vi "FPGA Main Default.vi"() -> ()   [LabVIEW 2019]
uses:
  Sub VIs/Utilities/Start Boolean.ctl
  <vilib>/Platform/TimedLoop/XDataNode/timing_clust.ctl
  <vilib>/Platform/TimedLoop/XDataNode/nitl_modes.ctl
  <vilib>/Platform/TimedLoop/XDataNode/wakeup.ctl
  Sub VIs/Utilities/SPI Configuration Group.ctl
  Sub VIs/Utilities/I2C Configuration Group.ctl
  Sub VIs/Utilities/PWM Configuration Group.ctl
  Sub VIs/Utilities/Encoder Configuration Group.ctl
  <vilib>/rvi/Emulation/niFpgaGetClockAttributes.vi
  <vilib>/rvi/Emulation/niFpgaSctlEmulationGetInTimedLoop.vi
  <vilib>/rvi/Emulation/niFpgaEmulationReportErrorSimple.vi
  <vilib>/rvi/Emulation/niFpgaEmulationIsFPGAContextNoSignature.vi
  <vilib>/rvi/errors/niFpgaSetErrorForExecOnDevCompSimple.vi
  <vilib>/rvi/eio/common/nirviEmuReportErrorAndStop.vi
  <vilib>/rvi/DataTransferAndStorage/Container/Common/niFpgaContainerGetUniqueNameForEmu.vi
  <vilib>/rvi/FIFO/Fifo_Resource/nirvififoEmulationSetSize.vi
  <vilib>/rvi/FIFO/Fifo_Resource/nirviFifoEmulationQueueMgr.vi
  <instcachedir>/0/nirviFifoEmulationQueueMgr_E5CAEC123FF24DC58D834DCA3CDAA9B5.lvgen/nirviFifoEmulationQueueMgr_E5CAEC123FF24DC58D834DCA3CDAA9B5_003.vi
  <vilib>/Utility/error.llb/Clear Errors.vi
  <vilib>/rvi/FIFO/Fifo_Resource/nirvififoEmulationCreateLock.vi
  <vilib>/rvi/Emulation/niFpgaProcessEmulError.vi
  <vilib>/rvi/FIFO/Fifo_Resource/nirvififoEmulationObtainLock.vi
  <vilib>/rvi/FIFO/Fifo_Resource/nirvififoEmulationReleaseLock.vi
  <vilib>/rvi/occurrence/nirviWaitOnOccurrenceBase.vi
  <vilib>/rvi/errors/nirviReportUnexpectedCaseInternalError.vi
  <vilib>/rvi/errors/nirviReportUnexpectedCaseInternalError (U32).vi
  <vilib>/rvi/FIFO/Fifo_Resource/nirvififoEmulationDetermineInputValidOut.vi
  <vilib>/rvi/Emulation/niFpgaCriticalErrorInLSC.vi
  <instcachedir>/0/nirviFifoEmulationQueueMgr_E5CAEC123FF24DC58D834DCA3CDAA9B5.lvgen/nirviFifoEmulationQueueMgr_E5CAEC123FF24DC58D834DCA3CDAA9B5_004.vi
  <instcachedir>/0/nirviFifoEmulationQueueMgr_E5CAEC123FF24DC58D834DCA3CDAA9B5.lvgen/nirviFifoEmulationQueueMgr_E5CAEC123FF24DC58D834DCA3CDAA9B5_005.vi
  <vilib>/rvi/eio/common/nirviEmuTemplateMethod_errors.vi
  <vilib>/rvi/interface/RandomDataEmulation/niFpgaRandomDataHandleErrors.vi
  Sub VIs/Utilities/ELVIS III Global.vi
  <vilib>/rvi/eio/common/nirviEmuTemplatePropertyGet_noerrors.vi
  <vilib>/rvi/eio/common/nirviEmuTemplatePropertySet_noerrors.vi
  <vilib>/rvi/Memory/Memory_Emulation/niFpgaMemoryEmulationCacheClearOnFirstRun.vi
  <vilib>/rvi/Memory/Memory_Emulation/nirvimemoryEmulationManagerCache_MakeExclusive.vi
  <vilib>/rvi/Memory/Memory_Emulation/niFpgaMemoryEmulationValidateCache.vi
  <vilib>/rvi/Memory/Memory_Emulation/nirvimemoryEmulationManagerCache_InsertValue.vi
  <vilib>/rvi/Memory/Memory_Emulation/nirvimemoryEmulationManagerCache_ReleaseExclusive.vi
  <vilib>/rvi/Memory/Memory_Emulation/nirvimemoryEmulationManagerCache_GetValue.vi
  <vilib>/rvi/Memory/Memory_Emulation/nirvimemoryEmulationManagerCache_SetValue.vi
  <vilib>/rvi/Memory/Memory_Emulation/nirvimemoryFastEmulation.vi
  <vilib>/rvi/Memory/Memory_Emulation/nirvimemoryEmulation.vi
  <vilib>/rvi/DataTransferAndStorage/Container/Common/niFpgaContainerSetEmuInfo.vi
  <vilib>/rvi/DataTransferAndStorage/Container/XNode/niFpgaContainer.xnode
  <vilib>/rvi/FIFO/Fifo_Resource/nirvififoEmulationRead.vi
  <vilib>/rvi/FIFO/Fifo_Resource/nirvififoEmulationWrite.vi
  <vilib>/Platform/TimedLoop/XDataNode/XDataNode.xnode
  <vilib>/eio/EIOMethodNode/EIOMethodNode.xnode
  <vilib>/LabVIEW Targets/FPGA/RIO/BlueMoonOnboardIO/nicrio_cRIO-BlueMoonOnboardAi_VoltageRange.ctl
  <vilib>/LabVIEW Targets/FPGA/RIO/BlueMoonOnboardIO/nicrio_cRIO-BlueMoonOnboardAi_TerminalMod.ctl
  <vilib>/rvi/interface/RandomDataEmulation/nirviRandomDataFpgaReadWriteTemplate.vi
  <vilib>/eio/EIOPropertyNode/EIOPropertyNode.xnode
  <vilib>/eio/EIONode/EIONode.xnode
  <vilib>/rvi/DataTransferAndStorage/Register/Emulation/niFpgaRegisterEmulation.vi
  <vilib>/rvi/LocalResourceManager/LocalResourceManager.xnode
  <vilib>/Platform/TimedLoop/XDataNode/XDNodeRunTimeDep.lvlib
  <vilib>/rvi/eio/common/nirviEmuTemplatePropertyGet_errors.vi
  <vilib>/rvi/eio/common/nirviEmuTemplatePropertySet_errors.vi
panel:
  in  "DATAGEN.B_1.CNTR":u32
  in  "DATAGEN.B_0.CNTR":u32
  in  "DATAGEN.A_1.CNTR":u32
  in  "DATAGEN.A_0.CNTR":u32
  in  "DATAGEN.ENA":fxp<+,4,4>
  in  "DATAGEN.A_0.FREQ_DIV":fxp<+,32,0>
  in  "DATAGEN.A_1.FREQ_DIV":fxp<+,32,0>
  in  "DATAGEN.B_1.FREQ_DIV":fxp<+,32,0>
  in  "DATAGEN.B_0.FREQ_DIV":fxp<+,32,0>
  out "DMA.SYS.RDY":bool
  out "AO.B.ELE_NUM":u32
  out "AO.A.ELE_NUM":u32
  in  "AO.B.SYNC":T1
  in  "AO.A.SYNC":T1
  in  "AO.SYNC":T1
  in  "SYNC":T1
  in  "B.SYNC":T1
  in  "A.SYNC":T1
  out "AI.A.STAT":u8
  out "AI.B.STAT":u8
  out "AI.DIFF_B_3.VAL":fxp<+/-,26,5>
  out "AI.DIFF_B_2.VAL":fxp<+/-,26,5>
  out "AI.DIFF_B_1.VAL":fxp<+/-,26,5>
  out "AI.DIFF_B_0.VAL":fxp<+/-,26,5>
  out "AI.B_7.VAL":fxp<+/-,26,5>
  out "AI.B_6.VAL":fxp<+/-,26,5>
  out "AI.B_5.VAL":fxp<+/-,26,5>
  out "AI.B_4.VAL":fxp<+/-,26,5>
  out "AI.B_3.VAL":fxp<+/-,26,5>
  out "AI.B_2.VAL":fxp<+/-,26,5>
  out "AI.B_1.VAL":fxp<+/-,26,5>
  out "AI.B_0.VAL":fxp<+/-,26,5>
  out "AI.DIFF_A_3.VAL":fxp<+/-,26,5>
  out "AI.DIFF_A_2.VAL":fxp<+/-,26,5>
  out "AI.DIFF_A_1.VAL":fxp<+/-,26,5>
  out "AI.DIFF_A_0.VAL":fxp<+/-,26,5>
  out "AI.A_7.VAL":fxp<+/-,26,5>
  out "AI.A_6.VAL":fxp<+/-,26,5>
  out "AI.A_5.VAL":fxp<+/-,26,5>
  out "AI.A_4.VAL":fxp<+/-,26,5>
  out "AI.A_3.VAL":fxp<+/-,26,5>
  out "AI.A_2.VAL":fxp<+/-,26,5>
  out "AI.A_1.VAL":fxp<+/-,26,5>
  out "AI.A_0.VAL":fxp<+/-,26,5>
  in  "UART.A.ENA":bool
  in  "UART.B.ENA":bool
  out "CONSOLE.ENA":bool
  in  "DO.LED3:0":u8 format="%04b"
  out "DI.BTN":u8 format="%08b"
  in  "IRQ.DI_BTN.ENA":bool
  in  "IRQ.DI_BTN.RISE":bool
  in  "IRQ.DI_BTN.FALL":bool
  in  "IRQ.DI_BTN.CNT":u32
  in  "IRQ.DI_BTN.NO":u8
  in  "IRQ.AI_A_1.NO":u8
  in  "IRQ.AI_A_0.NO":u8
  in  "IRQ.AI_A_1.THRESHOLD":fxp<+/-,26,5>
  in  "IRQ.AI_A_0.THRESHOLD":fxp<+/-,26,5>
  in  "IRQ.AI_A.CNFG":u8 format="%.0b"
  in  "IRQ.AI_A_0.HYSTERESIS":fxp<+/-,26,5>=15.999999523162842
  in  "IRQ.AI_A_1.HYSTERESIS":fxp<+/-,26,5>=15.999999523162842
  in  "IRQ.DIO_A_3.NO":u8
  in  "IRQ.DIO_A_2.NO":u8
  in  "IRQ.DIO_A_1.NO":u8
  in  "IRQ.DIO_A_0.NO":u8
  in  "IRQ.DIO_A_3.CNT":u32
  in  "IRQ.DIO_A_2.CNT":u32
  in  "IRQ.DIO_A_1.CNT":u32
  in  "IRQ.DIO_A_0.CNT":u32
  in  "IRQ.DIO_A_7:0.FALL":u8 format="%08b"
  in  "IRQ.DIO_A_7:0.RISE":u8 format="%08b"
  in  "IRQ.DIO_A_7:0.ENA":u8 format="%08b"
  in  "IRQ.TIMER.SETTIME":T1
  in  "IRQ.TIMER.WRITE":u32
  out "IRQ.TIMER.READ":u32
  out "UART.B.STAT":bool
  out "UART.A.STAT":bool
  out "AI.B.DMA_FULL":bool
  in  "AI.B.DMA_ENA":bool
  out "AI.B.VAL.RDY":bool
  in  "AI.B.CNFG":u8[](array[numeric])=[0, 1, 2, 3, 4, 5, 6, 7, 0, 0, 0, 0] format="%.0x"
  in  "AI.B.CNT":u8
  in  "AI.B.CNTR":u32=2000
  out "AO.B.DMA_IDL":bool
  in  "AO.B.DMA_CNTR":u32=200
  out "AO.A.DMA_IDL":bool
  in  "AO.A.DMA_CNTR":u32=200
  in  "AI.A.DMA_ENA":bool
  out "AI.A.DMA_FULL":bool
  out "AI.A.VAL.RDY":bool
  in  "AI.A.CNT":u8
  in  "AI.A.CNTR":u32=2000
  in  "AI.A.CNFG":u8[](array[numeric])=[0, 1, 2, 3, 4, 5, 6, 7, 0, 0, 0, 0] format="%.0x"
  in  "AO.B.DMA_ENA":fxp<+,2,2> format="%04b"
  out "AO.SYS.STAT":bool
  in  "AO.A.DMA_ENA":fxp<+,2,2> format="%04b"
  in  "AO.SYS.GO":T1
  in  "AO.B_0.VAL":fxp<+/-,20,5> format="%#_17g"
  in  "AO.B_1.VAL":fxp<+/-,20,5> format="%#_17g"
  in  "AO.A_0.VAL":fxp<+/-,20,5> format="%#_17g"
  in  "AO.A_1.VAL":fxp<+/-,20,5> format="%#_17g"
  in  "DIO.B_19:0.DIR":fxp<+,20,20> format="%.0b"
  in  "DO.B.DMA_CNTR":u16 format="%.0b"
  out "DIO.B_19:0.IN":fxp<+,20,20> format="%.0b"
  out "DI.B.DMA_IDL":bool
  in  "DIO.B_19:0.OUT":fxp<+,20,20> format="%.0b"
  out "DO.B.DMA_IDL":bool
  in  "DO.B.DMA_ENA":fxp<+,20,20> format="%020b"
  in  "DI.B.DMA_ENA":bool
  in  "DI.B.DMA_CNTR":u16 format="%.0b"
  in  "SYS.SELECTB":u64 format="%010x"
  out "ENC.B_0.CNTR":u32
  out "ENC.B_0.STAT":u8 format="%08b"
  in  "ENC.B_0.CNFG":u8
  in  "PWM.B_0.MAX":u16
  in  "PWM.B_0.CMP":u16
  in  "PWM.B_0.CNFG":u8 format="%08b"
  in  "PWM.B_0.CS":u8
  in  "PWM.B_1.MAX":u16
  in  "PWM.B_1.CMP":u16
  in  "PWM.B_1.CNFG":u8 format="%08b"
  in  "PWM.B_1.CS":u8
  out "PWM.B_0.CNTR":u16
  out "PWM.B_1.CNTR":u16
  in  "PWM.B_2.MAX":u16
  in  "PWM.B_2.CMP":u16
  in  "PWM.B_2.CNFG":u8 format="%08b"
  in  "PWM.B_2.CS":u8
  in  "PWM.B_3.MAX":u16
  in  "PWM.B_3.CMP":u16
  in  "PWM.B_3.CNFG":u8 format="%08b"
  in  "PWM.B_3.CS":u8
  in  "ENC.B_1.CNFG":u8
  out "ENC.B_1.CNTR":u32
  out "ENC.B_1.STAT":u8 format="%08b"
  out "PWM.B_2.CNTR":u16
  out "PWM.B_3.CNTR":u16
  in  "PWM.B_4.MAX":u16
  in  "PWM.B_4.CMP":u16
  in  "PWM.B_4.CNFG":u8 format="%08b"
  in  "PWM.B_4.CS":u8
  in  "PWM.B_5.MAX":u16
  in  "PWM.B_5.CMP":u16
  in  "PWM.B_5.CNFG":u8 format="%08b"
  in  "PWM.B_5.CS":u8
  in  "PWM.B_6.MAX":u16
  in  "PWM.B_6.CMP":u16
  in  "PWM.B_6.CNFG":u8 format="%08b"
  in  "PWM.B_6.CS":u8
  in  "PWM.B_7.MAX":u16
  in  "PWM.B_7.CMP":u16
  in  "PWM.B_7.CNFG":u8 format="%08b"
  in  "PWM.B_7.CS":u8
  out "ENC.B_2.CNTR":u32
  out "ENC.B_2.STAT":u8 format="%08b"
  out "PWM.B_4.CNTR":u16
  out "PWM.B_5.CNTR":u16
  out "PWM.B_6.CNTR":u16
  out "PWM.B_7.CNTR":u16
  out "ENC.B_3.CNTR":u32
  out "ENC.B_3.STAT":u8 format="%08b"
  in  "ENC.B_2.CNFG":u8
  in  "ENC.B_3.CNFG":u8
  out "SPI.B.STAT":u8 format="%08b"
  in  "SPI.B.GO":T1
  in  "SPI.B.CNT":u16=19
  in  "SPI.B.CNFG":u16=112
  out "SPI.B.DATI":u16
  in  "SPI.B.DATO":u16
  out "ENC.B_4.CNTR":u32
  out "ENC.B_4.STAT":u8 format="%08b"
  in  "ENC.B_4.CNFG":u8
  in  "PWM.B_8.MAX":u16
  in  "PWM.B_8.CMP":u16
  in  "PWM.B_8.CNFG":u8 format="%08b"
  in  "PWM.B_8.CS":u8
  in  "PWM.B_9.MAX":u16
  in  "PWM.B_9.CMP":u16
  in  "PWM.B_9.CNFG":u8 format="%08b"
  in  "PWM.B_9.CS":u8
  out "PWM.B_8.CNTR":u16
  out "PWM.B_9.CNTR":u16
  out "ENC.B_5.CNTR":u32
  out "ENC.B_5.STAT":u8 format="%08b"
  in  "ENC.B_5.CNFG":u8
  in  "PWM.B_10.MAX":u16
  in  "PWM.B_10.CMP":u16
  in  "PWM.B_10.CNFG":u8 format="%08b"
  in  "PWM.B_10.CS":u8
  in  "PWM.B_11.MAX":u16
  in  "PWM.B_11.CMP":u16
  in  "PWM.B_11.CNFG":u8 format="%08b"
  in  "PWM.B_11.CS":u8
  out "PWM.B_10.CNTR":u16
  out "PWM.B_11.CNTR":u16
  out "ENC.B_6.CNTR":u32
  out "ENC.B_6.STAT":u8 format="%08b"
  in  "ENC.B_6.CNFG":u8
  in  "PWM.B_12.MAX":u16
  in  "PWM.B_12.CMP":u16
  in  "PWM.B_12.CNFG":u8 format="%08b"
  in  "PWM.B_12.CS":u8
  in  "PWM.B_13.MAX":u16
  in  "PWM.B_13.CMP":u16
  in  "PWM.B_13.CNFG":u8 format="%08b"
  in  "PWM.B_13.CS":u8
  out "PWM.B_12.CNTR":u16
  out "PWM.B_13.CNTR":u16
  out "ENC.B_7.CNTR":u32
  out "ENC.B_7.STAT":u8 format="%08b"
  in  "ENC.B_7.CNFG":u8
  in  "PWM.B_14.MAX":u16
  in  "PWM.B_14.CMP":u16
  in  "PWM.B_14.CNFG":u8 format="%08b"
  in  "PWM.B_14.CS":u8
  in  "PWM.B_15.MAX":u16
  in  "PWM.B_15.CMP":u16
  in  "PWM.B_15.CNFG":u8 format="%08b"
  in  "PWM.B_15.CS":u8
  out "PWM.B_14.CNTR":u16
  out "PWM.B_15.CNTR":u16
  in  "I2C.B.GO":T1
  in  "I2C.B.CNFG":u8=1 format="%08b"
  in  "I2C.B.DATO":u8
  out "I2C.B.DATI":u8
  in  "I2C.B.ADDR":u8 format="%08b"
  in  "I2C.B.CNTR":u8=213
  in  "I2C.B.CNTL":u8 format="%08b"
  out "I2C.B.STAT":u8 format="%08b"
  out "ENC.B_8.CNTR":u32
  out "ENC.B_8.STAT":u8 format="%08b"
  in  "ENC.B_8.CNFG":u8
  in  "PWM.B_16.MAX":u16
  in  "PWM.B_16.CMP":u16
  in  "PWM.B_16.CNFG":u8 format="%08b"
  in  "PWM.B_16.CS":u8
  in  "PWM.B_17.MAX":u16
  in  "PWM.B_17.CMP":u16
  in  "PWM.B_17.CNFG":u8 format="%08b"
  in  "PWM.B_17.CS":u8
  out "PWM.B_16.CNTR":u16
  out "PWM.B_17.CNTR":u16
  out "ENC.B_9.CNTR":u32
  out "ENC.B_9.STAT":u8 format="%08b"
  in  "ENC.B_9.CNFG":u8
  in  "PWM.B_18.MAX":u16
  in  "PWM.B_18.CMP":u16
  in  "PWM.B_18.CNFG":u8 format="%08b"
  in  "PWM.B_18.CS":u8
  in  "PWM.B_19.MAX":u16
  in  "PWM.B_19.CMP":u16
  in  "PWM.B_19.CNFG":u8 format="%08b"
  in  "PWM.B_19.CS":u8
  out "PWM.B_18.CNTR":u16
  out "PWM.B_19.CNTR":u16
  out "ENC.A_9.CNTR":u32
  out "ENC.A_9.STAT":u8 format="%08b"
  in  "ENC.A_9.CNFG":u8
  in  "PWM.A_18.MAX":u16
  in  "PWM.A_18.CMP":u16
  in  "PWM.A_18.CNFG":u8 format="%08b"
  in  "PWM.A_18.CS":u8
  in  "PWM.A_19.MAX":u16
  in  "PWM.A_19.CMP":u16
  in  "PWM.A_19.CNFG":u8 format="%08b"
  in  "PWM.A_19.CS":u8
  out "PWM.A_18.CNTR":u16
  out "PWM.A_19.CNTR":u16
  out "ENC.A_8.CNTR":u32
  out "ENC.A_8.STAT":u8 format="%08b"
  in  "ENC.A_8.CNFG":u8
  in  "PWM.A_16.MAX":u16
  in  "PWM.A_16.CMP":u16
  in  "PWM.A_16.CNFG":u8 format="%08b"
  in  "PWM.A_16.CS":u8
  in  "PWM.A_17.MAX":u16
  in  "PWM.A_17.CMP":u16
  in  "PWM.A_17.CNFG":u8 format="%08b"
  in  "PWM.A_17.CS":u8
  out "PWM.A_16.CNTR":u16
  out "PWM.A_17.CNTR":u16
  out "I2C.A.STAT":u8 format="%08b"
  in  "I2C.A.CNTL":u8 format="%08b"
  in  "I2C.A.CNTR":u8=213
  in  "I2C.A.ADDR":u8 format="%08b"
  out "I2C.A.DATI":u8
  in  "I2C.A.DATO":u8
  in  "I2C.A.CNFG":u8=1 format="%08b"
  in  "I2C.A.GO":T1
  out "ENC.A_7.CNTR":u32
  out "ENC.A_7.STAT":u8 format="%08b"
  in  "ENC.A_7.CNFG":u8
  in  "PWM.A_14.MAX":u16
  in  "PWM.A_14.CMP":u16
  in  "PWM.A_14.CNFG":u8 format="%08b"
  in  "PWM.A_14.CS":u8
  in  "PWM.A_15.MAX":u16
  in  "PWM.A_15.CMP":u16
  in  "PWM.A_15.CNFG":u8 format="%08b"
  in  "PWM.A_15.CS":u8
  out "PWM.A_14.CNTR":u16
  out "PWM.A_15.CNTR":u16
  out "ENC.A_6.CNTR":u32
  out "ENC.A_6.STAT":u8 format="%08b"
  in  "ENC.A_6.CNFG":u8
  in  "PWM.A_12.MAX":u16
  in  "PWM.A_12.CMP":u16
  in  "PWM.A_12.CNFG":u8 format="%08b"
  in  "PWM.A_12.CS":u8
  in  "PWM.A_13.MAX":u16
  in  "PWM.A_13.CMP":u16
  in  "PWM.A_13.CNFG":u8 format="%08b"
  in  "PWM.A_13.CS":u8
  out "PWM.A_12.CNTR":u16
  out "PWM.A_13.CNTR":u16
  out "ENC.A_5.CNTR":u32
  out "ENC.A_5.STAT":u8 format="%08b"
  in  "ENC.A_5.CNFG":u8
  in  "PWM.A_10.MAX":u16
  in  "PWM.A_10.CMP":u16
  in  "PWM.A_10.CNFG":u8 format="%08b"
  in  "PWM.A_10.CS":u8
  in  "PWM.A_11.MAX":u16
  in  "PWM.A_11.CMP":u16
  in  "PWM.A_11.CNFG":u8 format="%08b"
  in  "PWM.A_11.CS":u8
  out "PWM.A_10.CNTR":u16
  out "PWM.A_11.CNTR":u16
  out "ENC.A_4.CNTR":u32
  out "ENC.A_4.STAT":u8 format="%08b"
  in  "ENC.A_4.CNFG":u8
  in  "PWM.A_8.MAX":u16
  in  "PWM.A_8.CMP":u16
  in  "PWM.A_8.CNFG":u8 format="%08b"
  in  "PWM.A_8.CS":u8
  in  "PWM.A_9.MAX":u16
  in  "PWM.A_9.CMP":u16
  in  "PWM.A_9.CNFG":u8 format="%08b"
  in  "PWM.A_9.CS":u8
  out "PWM.A_8.CNTR":u16
  out "PWM.A_9.CNTR":u16
  in  "SPI.A.DATO":u16
  out "SPI.A.DATI":u16
  in  "SPI.A.CNFG":u16=112
  in  "SPI.A.CNT":u16=19
  in  "SPI.A.GO":T1
  out "SPI.A.STAT":u8 format="%08b"
  in  "ENC.A_3.CNFG":u8
  in  "ENC.A_2.CNFG":u8
  out "ENC.A_3.CNTR":u32
  out "ENC.A_3.STAT":u8 format="%08b"
  out "PWM.A_6.CNTR":u16
  out "PWM.A_7.CNTR":u16
  out "ENC.A_2.CNTR":u32
  out "ENC.A_2.STAT":u8 format="%08b"
  out "PWM.A_4.CNTR":u16
  out "PWM.A_5.CNTR":u16
  in  "PWM.A_6.MAX":u16
  in  "PWM.A_6.CMP":u16
  in  "PWM.A_6.CNFG":u8 format="%08b"
  in  "PWM.A_6.CS":u8
  in  "PWM.A_7.MAX":u16
  in  "PWM.A_7.CMP":u16
  in  "PWM.A_7.CNFG":u8 format="%08b"
  in  "PWM.A_7.CS":u8
  in  "PWM.A_4.MAX":u16
  in  "PWM.A_4.CMP":u16
  in  "PWM.A_4.CNFG":u8 format="%08b"
  in  "PWM.A_4.CS":u8
  in  "PWM.A_5.MAX":u16
  in  "PWM.A_5.CMP":u16
  in  "PWM.A_5.CNFG":u8 format="%08b"
  in  "PWM.A_5.CS":u8
  out "PWM.A_3.CNTR":u16
  out "PWM.A_2.CNTR":u16
  out "ENC.A_1.STAT":u8 format="%08b"
  out "ENC.A_1.CNTR":u32
  in  "ENC.A_1.CNFG":u8
  in  "PWM.A_3.CS":u8
  in  "PWM.A_3.CNFG":u8 format="%08b"
  in  "PWM.A_3.CMP":u16
  in  "PWM.A_3.MAX":u16
  in  "PWM.A_2.CS":u8
  in  "PWM.A_2.CNFG":u8 format="%08b"
  in  "PWM.A_2.CMP":u16
  in  "PWM.A_2.MAX":u16
  out "ENC.A_0.STAT":u8 format="%08b"
  out "ENC.A_0.CNTR":u32
  in  "ENC.A_0.CNFG":u8
  in  "PWM.A_1.MAX":u16
  in  "PWM.A_1.CMP":u16
  in  "PWM.A_1.CNFG":u8 format="%08b"
  in  "PWM.A_1.CS":u8
  out "PWM.A_1.CNTR":u16
  out "PWM.A_0.CNTR":u16
  in  "PWM.A_0.CS":u8
  in  "PWM.A_0.CNFG":u8 format="%08b"
  in  "PWM.A_0.CMP":u16
  in  "PWM.A_0.MAX":u16
  in  "SYS.SELECTA":u64 format="%010x"
  in  "DI.A.DMA_CNTR":u16 format="%.0b"
  in  "DI.A.DMA_ENA":bool
  in  "DO.A.DMA_ENA":fxp<+,20,20> format="%020b"
  out "DO.A.DMA_IDL":bool
  in  "DIO.A_19:0.OUT":fxp<+,20,20> format="%.0b"
  out "DI.A.DMA_IDL":bool
  out "DIO.A_19:0.IN":fxp<+,20,20> format="%.0b"
  in  "DO.A.DMA_CNTR":u16 format="%.0b"
  in  "DIO.A_19:0.DIR":fxp<+,20,20> format="%.0b"
  # "Connector B"
  # "System"
  # "Onboard Devices"
  # "Connector A"
  # "Buttons & LEDs"
  # "Digital I/O"
  # "PWM"
  # "Encoder"
  # "SPI Master"
  # "Analog Out"
  # "Analog In"
  # "Digital Interrupt"
  # "Digital I/O"
  # "PWM"
  # "Encoder"
  # "SPI Master"
  # "Analog Out"
  # "Analog In"
  # "Button Interrupt"
  # "Block Write AO"
  # "Block Write AO"
  # "Block Read DI"
  # "Block Read DI"
  # "I2C Master"
  # "I2C Master"
  # "Block Write DO"
  # "Block Write DO"
  # "Timer Interrupt"
  # "Data Generator"
  # "Data Generator"
  # "Analog Interrupt"
  # "IO Configuration"
  # "Console Output"
  # "IO Configuration"
  # "UART"
  # "UART"
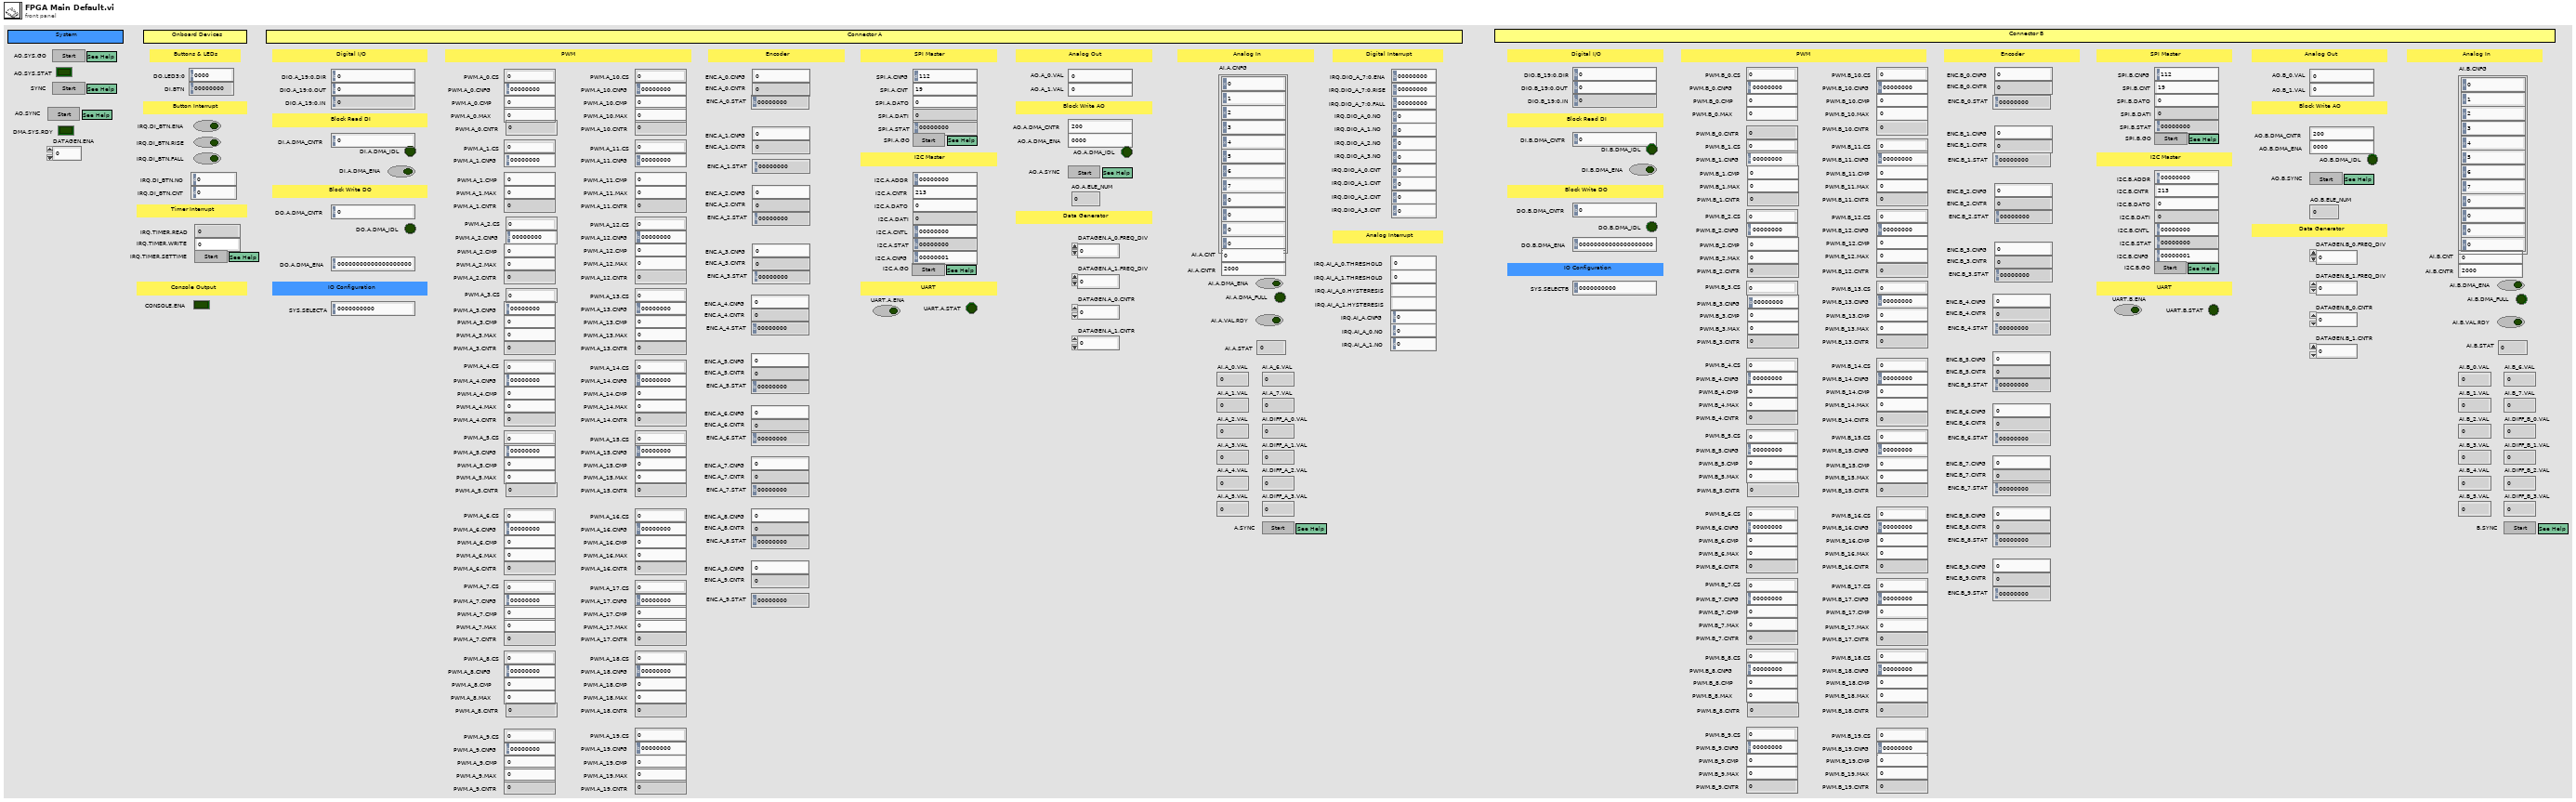
[diagram p1: front panel]
types:
  T1 = typedef "Start Boolean.ctl" = bool
  T2 = typedef "XDNodeRunTimeDep.lvlib/timing_clust.ctl" = cluster{"Expected End [f-1]":u64, "Actual End [f-1]":u64, "Finished Late? [f-1]":bool, "Expected End [i-1]":u64, "Actual End [i-1]":u64, "Finished Late? [i-1]":bool, "Expected Start [i]":u64, "Actual Start [i]":u64, "Expected Start [f]":u64, "Actual Start [f]":u64, "Source Name":string, "Structure Name":string, "Period":i64, "Deadline":i64, "Offset":i64, "Start":i64, "Priority":i32, "Timeout":i32, "Mode":T3, "Wakeup Reason":T4, "Error":errorcluster, "Source Type":string, "Secondary Source Type":string, "Global End Time":u64, "Global Start Time":u64, "Frame Duration":u64, "Iteration Duration":u64, "Assigned CPU":i32, "I/O Scan Engine Mode":u32}
  T3 = typedef "XDNodeRunTimeDep.lvlib/nitl_modes.ctl" = enum32{"No Change", "Process missed periods, maintain original phase", "Discard missed periods, maintain original phase", "Process missed periods, ignore original phase", "Discard missed periods, ignore original phase"}
  T4 = typedef "XDNodeRunTimeDep.lvlib/wakeup.ctl" = enum32{"Normal", "Aborted", "Asynchronous wakeup", "Timing source error", "Timed loop error", "Timeout"}
  T5 = typedef "Encoder Configuration Group.ctl" = cluster{"ENC.CNFG":u8, "ENC.CNTR":u32, "ENC.STAT":u8}
  T6 = typedef "PWM Configuration Group.ctl" = cluster{"PWM.0.CS":u8, "PWM.0.CNFG":u8, "PWM.0.CMP":u16, "PWM.0.MAX":u16, "PWM.0.CNTR":u16, "PWM.1.CS":u8, "PWM.1.CNFG":u8, "PWM.1.CMP":u16, "PWM.1.MAX":u16, "PWM.1.CNTR":u16}
  T7 = typedef "I2C Configuration Group.ctl" = cluster{"I2C.GO":T1, "I2C.CNFG":u8, "I2C.DATO":u8, "I2C.DATI":u8, "I2C.ADDR":u8, "I2C.CNTR":u8, "I2C.CNTL":u8, "I2C.STAT":u8}
  T8 = typedef "SPI Configuration Group.ctl" = cluster{"SPI.STAT":u8, "SPI.GO":T1, "SPI.CNT":u16, "SPI.CNFG":u16, "SPI.DATI":u16, "SPI.DATO":u16}
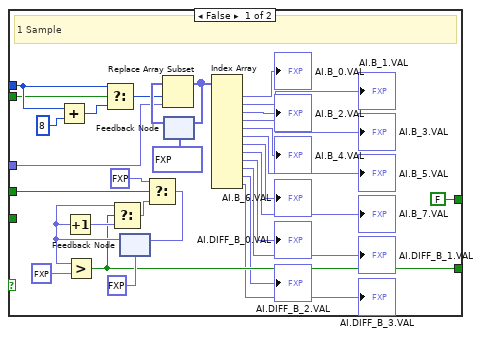
[diagram p15: hidden frame]
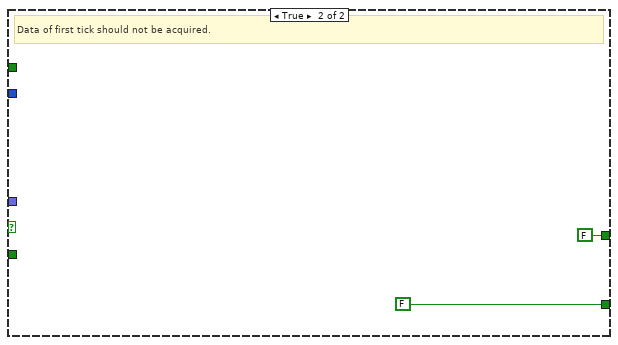
[diagram p16: hidden frame]
diagram:
  w3 = u32 0  # Address
  w4 = u32 0  # Address
  w5 = u32 0  # Address
  w6 = u32 0  # Address
  # "The Timed Loop does not allow writing the same FIFO outside the Timed Loop. Use another FIFO to push all interrupts from Button in the Timed Loop to the IRQ Queue."
  # "The FPGA timer fires the interrupt request (IRQ) when TIMER.Read counts down to zero. If TIMER.Read is not zero, it counts down to one per microsecond."
  # "The analog output nodes take some time before the FPGA write the values to the pins. The GO and STAT registers are used to handshake between the FPGA and host. When the host wants the values to be written, the host sets the GO register to TRUE. If the host reads the STAT register before setting the value of the GO register, it can wait for the value of the STAT register to invert. The value inversion tells the host that the output values have been written."
  # "The only interface that sends interrupts to the RT side. Timer interrupts, analog input interrupts, digital input interrupts, and SPI interrupt share this interface.\n\nAll interrupts work in sequence. One interrupt waits until the previous interrupt request (IRQ) gets acknowledged on the RT side."
  # "Because Write Finished Queue cannot be shared between a single-cycle Timed Loop and any other loop, Digital Write Finished Queue is required. Use this queue to transfer IRQ from DIO to IRQ Write Finished Queue."
  n1 = node-c288() -> (w8:T2)  [unwired: 1 in]
  n2 = while {
    stop <- FALSE stop-if-true
    # "Send Write Finished IRQ to RT"
    n3 = xnode ("FIFO Method Node")("超时"=-1 ("Timeout")) -> ("元素"=w25:u8)  [unwired: 1 in, 2 out]
    n4 = call <vilib>:"niFPGA Interrupt.vi"("Wait Until Cleared (F)"=TRUE, "IRQ Number (0)"=w25) -> ()  [unwired: 1 in]
  }
  n5 = timed-loop {
    timing: w8 -> [_]
    timing-out: [_] -> w7
    i -> [w29]
    stop <- _ stop-if-true
    # "DMA initialization needs 0.5s"
    n6 = Greater?(x=w29, y=20000000) -> (0:→"DMA.SYS.RDY":bool)
  }
  n7 = node-c288(w7) -> ()
  n8 = while {
    stop <- FALSE stop-if-true
    # "Timer"
    n9 = flat-sequence {
      frame #0 {
        n10 = call "Loop Timer6"("Count(uSec)"=u8 1 ("Count(mSec)")) -> ()  [unwired: 1 out]
      }
      frame #1 {
        n11 = feedback #1(u32 0 ("Timeout")) -> (w35:u32)
        n12 = Select(t="IRQ.TIMER.WRITE", s="IRQ.TIMER.SETTIME", f=w35) -> (s? t:f=w37:u32)
        n13 = case shown="默认" w37 {
          selector: w37 -> [w40 w43]
          tunnel: [w40 w41] -> w36
          frame 0 {
          }
          frame Default {
            n14 = Decrement(x=w43) -> (x-1=w42:u32)
            n15 = case shown="0" w42 {
              selector: w42 -> [w44 w47]
              tunnel: [w44 w47] -> w41
              frame Default {
              }
              frame 0 {
                n16 = global read "ELVIS III Global.vi" "Timer.IRQ_NO"() -> (w45:u8)
                n17 = xnode ("FIFO Method Node")("元素"=w45, "超时"=-1 ("Timeout")) -> ()  [unwired: 1 in, 2 out]
              }
            }
          }
        }
        "IRQ.TIMER.READ" <- w36
        n18 = feedback-in #1(w36) -> ()
      }
    }
  }
  n19 = while {
    stop <- FALSE stop-if-true
    # "DO Bank A Block Write Finished IRQ"
    n20 = feedback #2(u8 0 ("Element")) -> (w52:u8)
    n21 = feedback #3(FALSE ("Timed Out?")) -> (w54:bool)
    n22 = case shown="假" w54 {
      tunnel: [w56 w58] -> w48
      tunnel: w52 -> [_ w58]
      frame False {
        n23 = xnode ("FIFO Method Node")("超时"=-1 ("Timeout")) -> ("元素"=w56:u8)  [unwired: 1 in, 2 out]
      }
      frame True {
      }
    }
    n24 = feedback-in #2(w48) -> ()
    n25 = xnode ("FIFO Method Node")("元素"=w48, "超时"=0 ("Timeout")) -> ("超时？"=w49:bool)  [unwired: 1 in, 1 out]
    n26 = feedback-in #3(w49) -> ()
  }
  n27 = while {
    stop <- FALSE stop-if-true
    # "DO Bank B Block Write Finished IRQ"
    n28 = feedback #4(u8 0 ("Element")) -> (w63:u8)
    n29 = feedback #5(FALSE ("Timed Out?")) -> (w65:bool)
    n30 = case shown="假" w65 {
      tunnel: [w67 w69] -> w59
      tunnel: w63 -> [_ w69]
      frame False {
        n31 = xnode ("FIFO Method Node")("超时"=-1 ("Timeout")) -> ("元素"=w67:u8)  [unwired: 1 in, 2 out]
      }
      frame True {
      }
    }
    n32 = feedback-in #4(w59) -> ()
    n33 = xnode ("FIFO Method Node")("元素"=w59, "超时"=0 ("Timeout")) -> ("超时？"=w60:bool)  [unwired: 1 in, 1 out]
    n34 = feedback-in #5(w60) -> ()
  }
  n35 = xnode "VI-Defined FIFO Configuration"() -> ("FIFO输出"=w18:refnum<k21>)
  n36 = xnode "VI-Defined FIFO Configuration"() -> ()  [unwired: 1 out]
  n37 = node-c288() -> (w13:T2)  [unwired: 1 in]
  n38 = while {
    stop <- FALSE stop-if-true
    # "A/AI Read Input"
    n39 = xnode ("FIFO Read")("超时"=-1 ("Timeout")) -> ("元素"=w82:u16)  [unwired: 1 in, 2 out]
    n40 = node-c288() -> (w71:T2)
    n41 = timed-loop {
      timing: w71 -> [_]
      timing-out: [_] -> w70
      tunnel: w82 -> [w100]
      tunnel: [w94] -> w79
      tunnel: [w90] -> w78
      tunnel: [w89] -> w77
      tunnel: [w88] -> w76
      tunnel: [w87] -> w73
      stop <- TRUE stop-if-true
      n42 = Number To Boolean Array(number=w100) -> (Boolean array=w99:bool[])
      n43 = Index Array(array=w99, index #7=7 ("index")) -> (element #1=w98:bool, element #2=w97:bool, element #3=w96:bool, element #4=w88:bool, element #5=w92:bool, element #6=w91:bool, element #7=w87:bool)  [unwired: 6 in]
      n44 = Build Array(w98, w97, w96) -> (w95:bool[])
      n45 = Build Array(w92, w91) -> (w93:bool[])
      n46 = Boolean Array To Number(Boolean array=w95) -> (number=w89:u8)
      n47 = Boolean To (0,1)(Boolean=w88) -> (0, 1=w94:i16)
      n48 = Boolean Array To Number(Boolean array=w93) -> (number=w90:u8)
    }
    n49 = node-c288(w70) -> ()
    n50 = xnode "FPGA I/O Method Node"("Voltage Range [i + 1]"=w78, "Terminal Mode [i + 1]"=w79, "Channel Number [i + 1]"=w77) -> ("Data [i]"=w74:fxp<+/-,24,5>)  [unwired: 1 in, 1 out]
    n51 = feedback-in #6(w76) -> ()
    n52 = feedback #6() -> (w72:bool)  [unwired: 1 in]
    n53 = feedback #7() -> (w75:u8)  [unwired: 1 in]
    n54 = feedback-in #7(w77) -> ()
    n55 = node-c288() -> (w81:T2)  [unwired: 1 in]
    n56 = timed-loop {
      timing: w81 -> [_]
      timing-out: [_] -> w80
      tunnel: w74 -> [w112]
      tunnel: w73 -> [w107]
      tunnel: w75 -> [w110]
      tunnel: w72 -> [w109]
      stop <- TRUE stop-if-true
      n57 = feedback #8() -> (w105:bool)  [unwired: 1 in]
      n58 = case shown="假" w107 {
        selector: w107 -> [w115 _]
        tunnel: w112 -> [w120 _]
        tunnel: w110 -> [w119 _]
        tunnel: w109 -> [w118 _]
        tunnel: [w116 FALSE] -> w108
        tunnel: [w114 FALSE ("Timed Out?")] -> w106
        tunnel: w105 -> [w113 _]
        frame False {
          # "Data after first tick"
          n59 = case shown="假" "AI.A.DMA_ENA" {
            tunnel: w120 -> [w149 w157]
            tunnel: w119 -> [w137 _]
            tunnel: w115 -> [w140 _]
            tunnel: w118 -> [w136 _]
            tunnel: [w135 FALSE] -> w116
            tunnel: [FALSE ("Timed Out?") w152] -> w114
            tunnel: w113 -> [_ w153]
            frame False {
              # "1 Sample"
              n60 = Add(x=w137, y=u8 8) -> (x+y=w147:u8)
              n61 = Select(t=w137, s=w136, f=w147) -> (s? t:f=w146:u8)
              n62 = feedback #9(fxp<+,4,4> 0.0 ("y")) -> (w141:fxp<+,4,4>)
              n63 = Increment(x=w141) -> (x+1=w143:fxp<+,4,4>)
              n64 = Greater?(x=w141, y=fxp<+,4,4> 11.0) -> (0:w135:bool)
              n65 = Select(t=w141, s=w135, f=w143) -> (s? t:f=w142:fxp<+,4,4>)
              n66 = Select(t=fxp<+,4,4> 0.0 ("y"), s=w140, f=w142) -> (s? t:f=w145:fxp<+,4,4>)
              n67 = feedback-in #9(w145) -> ()
              n68 = feedback #10(fxp<+/-,26,5>[] [0.0, 0.0, 0.0, 0.0, 0.0, 0.0, 0.0, 0.0, 0.0, 0.0, 0.0, 0.0] ("Array")) -> (w150:fxp<+/-,26,5>[])
              n69 = Replace Array Subset(array=w150, new element=w149, index=w146) -> (w134:fxp<+/-,26,5>[])
              n70 = feedback-in #10(w134) -> ()
              n71 = Index Array(array=w134) -> (element #1=→"AI.A_0.VAL":fxp<+/-,26,5>, element #2=→"AI.A_1.VAL":fxp<+/-,26,5>, element #3=→"AI.A_2.VAL":fxp<+/-,26,5>, element #4=→"AI.A_3.VAL":fxp<+/-,26,5>, element #5=→"AI.A_4.VAL":fxp<+/-,26,5>, element #6=→"AI.A_5.VAL":fxp<+/-,26,5>, element #7=→"AI.A_6.VAL":fxp<+/-,26,5>, element #8=→"AI.A_7.VAL":fxp<+/-,26,5>, element #9=→"AI.DIFF_A_0.VAL":fxp<+/-,26,5>, element #10=→"AI.DIFF_A_1.VAL":fxp<+/-,26,5>, element #11=→"AI.DIFF_A_2.VAL":fxp<+/-,26,5>, element #12=→"AI.DIFF_A_3.VAL":fxp<+/-,26,5>)  [unwired: 12 in]
            }
            frame True {
              # "N Sample"
              n72 = xnode ("FIFO Write")("元素"=w157, "超时"=0 ("Timeout")) -> ("超时？"=w154:bool)  [unwired: 1 in, 1 out]
              n73 = Or(x=w154, y=w153) -> (x .or. y?=w152:bool)
            }
          }
        }
        frame True {
          # "Data of first tick should not be acquired."
        }
      }
      "AI.A.VAL.RDY" <- w108
      "AI.A.DMA_FULL" <- w106
      n74 = feedback-in #8(w106) -> ()
    }
    n75 = node-c288(w80) -> ()
  }
  n76 = while {
    tunnel: w18 -> [w167]
    stop <- FALSE stop-if-true
    # "AI IRQ for 1 Sample"
    n77 = local read "AI.A_0.VAL"() -> (w165:fxp<+/-,26,5>)
    n78 = local read "AI.A_1.VAL"() -> (w164:fxp<+/-,26,5>)
    n79 = Number To Boolean Array(number="IRQ.AI_A.CNFG") -> (Boolean array=w179:bool[])
    n80 = Index Array(array=w179) -> (element #1=w173:bool, element #2=w172:bool, element #3=w171:bool, element #4=w170:bool)  [unwired: 4 in]
    n81 = call "ELVIS III Check AI IRQ (FXP).vi"("Hysteresis"="IRQ.AI_A_1.HYSTERESIS", "FIFO In"=w167, "IRQ Number"="IRQ.AI_A_1.NO", "Threshold"="IRQ.AI_A_1.THRESHOLD", "Analog Value"=w164, "Rising Edge?"=w170, "Enable Interrupt?"=w171) -> ()  [unwired: 5 in]
    n82 = call "ELVIS III Check AI IRQ (FXP).vi"("Hysteresis"="IRQ.AI_A_0.HYSTERESIS", "FIFO In"=w167, "IRQ Number"="IRQ.AI_A_0.NO", "Threshold"="IRQ.AI_A_0.THRESHOLD", "Analog Value"=w165, "Rising Edge?"=w172, "Enable Interrupt?"=w173) -> ()  [unwired: 5 in]
  }
  n83 = Generate Occurrence() -> (w14:refnum<k4>)
  n84 = while {
    tunnel: w14 -> [w182]
    stop <- FALSE stop-if-true
    # "A/AI Generate Configurations"
    n85 = node-c288() -> (w189:T2)  [unwired: 1 in]
    n86 = timed-loop {
      timing: w189 -> [_]
      timing-out: [_] -> w188
      tunnel: ["AI.A.CNTR"] -> w185
      tunnel: ["AI.A.CNFG"] -> w187
      tunnel: [w233] -> w186
      tunnel: ["AI.A.CNT"] -> w184
      stop <- TRUE stop-if-true
      n87 = feedback-in #11("AI.A.CNFG") -> ()
      n88 = feedback #11() -> (w231:u8[])  [unwired: 1 in]
      n89 = feedback-in #12("AI.A.CNT") -> ()
      n90 = feedback #12() -> (w235:u8)  [unwired: 1 in]
      n91 = call "Check If Arrays Equal.vi"("y"="AI.A.CNFG", "x"=w231) -> ("x != y?"=w229:bool)  [unwired: 4 in]
      n92 = Not Equal?(x=w235, y="AI.A.CNT") -> (x != y?=w234:bool)
      n93 = Or(x=w229, y=w234) -> (x .or. y?=w233:bool)
    }
    n94 = node-c288(w188) -> ()
    n95 = case shown="真" "A.SYNC" {
      tunnel: w182 -> [_ w226]
      tunnel: w186 -> [w223 _]
      tunnel: [w223 TRUE] -> w183
      frame False {
      }
      frame True {
        n96 = Wait on Occurrence(2:w226, 3:10000 ("ms timeout (-1)")) -> ()  [unwired: 1 in, 1 out]
      }
    }
    n97 = for {
      N: w184 -> [_]
      tunnel: w187 -> [w194] mode=indexing
      tunnel: w185 -> [w192]
      tunnel: w183 -> [w193]
      shift-right: [w191] -> w180
      shift-left: w184 -> [w191]
      i -> [w198]
      n98 = flat-sequence {
        tunnel: w198 -> [w200]
        tunnel: w193 -> [w201]
        tunnel: w194 -> [w202]
        tunnel: [w202] -> w197
        tunnel: [w201] -> w196
        tunnel: [w200] -> w195
        tunnel: w192 -> [w199]
        tunnel: w197 -> [w205]
        tunnel: w196 -> [w207]
        tunnel: w195 -> [w206]
        frame #0 {
          n99 = call "Loop Timer"("Count(Ticks)"=w199) -> ()  [unwired: 1 out]
        }
        frame #1 {
          n100 = node-c288() -> (w204:T2)  [unwired: 1 in]
          n101 = timed-loop {
            timing: w204 -> [_]
            timing-out: [_] -> w203
            tunnel: w207 -> [w218]
            tunnel: w206 -> [w217]
            tunnel: w205 -> [w215]
            stop <- TRUE stop-if-true
            n102 = Equal To 0?(x=w217) -> (x = 0?=w212:bool)
            n103 = Number To Boolean Array(number=w215) -> (Boolean array=w210:bool[])
            n104 = And(x=w218, y=w212) -> (x .and. y?=w211:bool)
            n105 = Replace Array Subset(array=w210, new element=w211, index=7) -> (w213:bool[])
            n106 = Boolean Array To Number(Boolean array=w213) -> (number=w214:u16)
            n107 = xnode ("FIFO Write")("元素"=w214, "超时"=0 ("Timeout")) -> ()  [unwired: 1 in, 2 out]
          }
          n108 = node-c288(w203) -> ()
        }
      }
    }
    "AI.A.STAT" <- w180
  }
  n109 = timed-loop {
    tunnel: w14 -> [w242]
    timing: w13 -> [_]
    timing-out: [_] -> w12
    stop <- FALSE stop-if-true
    n110 = case shown="真" "SYNC" {
      tunnel: w242 -> [_ w243]
      frame False {
      }
      frame True {
        n111 = Set Occurrence(w243) -> ()
      }
    }
  }
  n112 = node-c288(w12) -> ()
  n113 = xnode "VI-Defined FIFO Configuration"() -> ()  [unwired: 1 out]
  n114 = while {
    tunnel: w14 -> [w248]
    stop <- FALSE stop-if-true
    # "B/AI Generate Configurations"
    n115 = node-c288() -> (w255:T2)  [unwired: 1 in]
    n116 = timed-loop {
      timing: w255 -> [_]
      timing-out: [_] -> w254
      tunnel: ["AI.B.CNTR"] -> w251
      tunnel: ["AI.B.CNFG"] -> w253
      tunnel: [w299] -> w252
      tunnel: ["AI.B.CNT"] -> w250
      stop <- TRUE stop-if-true
      n117 = feedback-in #13("AI.B.CNFG") -> ()
      n118 = feedback #13() -> (w297:u8[])  [unwired: 1 in]
      n119 = feedback-in #14("AI.B.CNT") -> ()
      n120 = feedback #14() -> (w301:u8)  [unwired: 1 in]
      n121 = call "Check If Arrays Equal.vi"("y"="AI.B.CNFG", "x"=w297) -> ("x != y?"=w295:bool)  [unwired: 4 in]
      n122 = Not Equal?(x=w301, y="AI.B.CNT") -> (x != y?=w300:bool)
      n123 = Or(x=w295, y=w300) -> (x .or. y?=w299:bool)
    }
    n124 = node-c288(w254) -> ()
    n125 = case shown="真" "B.SYNC" {
      tunnel: w248 -> [_ w292]
      tunnel: w252 -> [w289 _]
      tunnel: [w289 TRUE] -> w249
      frame False {
      }
      frame True {
        n126 = Wait on Occurrence(2:w292, 3:10000 ("ms timeout (-1)")) -> ()  [unwired: 1 in, 1 out]
      }
    }
    n127 = for {
      N: w250 -> [_]
      tunnel: w253 -> [w260] mode=indexing
      tunnel: w251 -> [w258]
      tunnel: w249 -> [w259]
      shift-right: [w257] -> w246
      shift-left: w250 -> [w257]
      i -> [w264]
      n128 = flat-sequence {
        tunnel: w264 -> [w266]
        tunnel: w259 -> [w267]
        tunnel: w260 -> [w268]
        tunnel: [w268] -> w263
        tunnel: [w267] -> w262
        tunnel: [w266] -> w261
        tunnel: w258 -> [w265]
        tunnel: w263 -> [w271]
        tunnel: w262 -> [w273]
        tunnel: w261 -> [w272]
        frame #0 {
          n129 = call "Loop Timer5"("Count(Ticks)"=w265) -> ()  [unwired: 1 out]
        }
        frame #1 {
          n130 = node-c288() -> (w270:T2)  [unwired: 1 in]
          n131 = timed-loop {
            timing: w270 -> [_]
            timing-out: [_] -> w269
            tunnel: w273 -> [w284]
            tunnel: w272 -> [w283]
            tunnel: w271 -> [w281]
            stop <- TRUE stop-if-true
            n132 = Equal To 0?(x=w283) -> (x = 0?=w278:bool)
            n133 = Number To Boolean Array(number=w281) -> (Boolean array=w276:bool[])
            n134 = And(x=w284, y=w278) -> (x .and. y?=w277:bool)
            n135 = Replace Array Subset(array=w276, new element=w277, index=7) -> (w279:bool[])
            n136 = Boolean Array To Number(Boolean array=w279) -> (number=w280:u16)
            n137 = xnode ("FIFO Write")("元素"=w280, "超时"=0 ("Timeout")) -> ()  [unwired: 1 in, 2 out]
          }
          n138 = node-c288(w269) -> ()
        }
      }
    }
    "AI.B.STAT" <- w246
  }
  n139 = while {
    stop <- FALSE stop-if-true
    # "B/AI Read Input"
    n140 = xnode ("FIFO Read")("超时"=-1 ("Timeout")) -> ("元素"=w318:u16)  [unwired: 1 in, 2 out]
    n141 = node-c288() -> (w307:T2)
    n142 = timed-loop {
      timing: w307 -> [_]
      timing-out: [_] -> w306
      tunnel: w318 -> [w336]
      tunnel: [w330] -> w315
      tunnel: [w326] -> w314
      tunnel: [w325] -> w313
      tunnel: [w324] -> w312
      tunnel: [w323] -> w309
      stop <- TRUE stop-if-true
      n143 = Number To Boolean Array(number=w336) -> (Boolean array=w335:bool[])
      n144 = Index Array(array=w335, index #7=7 ("index")) -> (element #1=w334:bool, element #2=w333:bool, element #3=w332:bool, element #4=w324:bool, element #5=w328:bool, element #6=w327:bool, element #7=w323:bool)  [unwired: 6 in]
      n145 = Build Array(w334, w333, w332) -> (w331:bool[])
      n146 = Build Array(w328, w327) -> (w329:bool[])
      n147 = Boolean Array To Number(Boolean array=w331) -> (number=w325:u8)
      n148 = Boolean To (0,1)(Boolean=w324) -> (0, 1=w330:i16)
      n149 = Boolean Array To Number(Boolean array=w329) -> (number=w326:u8)
    }
    n150 = node-c288(w306) -> ()
    n151 = xnode "FPGA I/O Method Node"("Voltage Range [i + 1]"=w314, "Terminal Mode [i + 1]"=w315, "Channel Number [i + 1]"=w313) -> ("Data [i]"=w310:fxp<+/-,24,5>)  [unwired: 1 in, 1 out]
    n152 = feedback-in #15(w312) -> ()
    n153 = feedback #15() -> (w308:bool)  [unwired: 1 in]
    n154 = feedback #16() -> (w311:u8)  [unwired: 1 in]
    n155 = feedback-in #16(w313) -> ()
    n156 = node-c288() -> (w317:T2)  [unwired: 1 in]
    n157 = timed-loop {
      timing: w317 -> [_]
      timing-out: [_] -> w316
      tunnel: w310 -> [w348]
      tunnel: w309 -> [w343]
      tunnel: w311 -> [w346]
      tunnel: w308 -> [w345]
      stop <- TRUE stop-if-true
      n158 = feedback #17() -> (w341:bool)  [unwired: 1 in]
      n159 = case shown="假" w343 {
        selector: w343 -> [w351 _]
        tunnel: w348 -> [w356 _]
        tunnel: w346 -> [w355 _]
        tunnel: w345 -> [w354 _]
        tunnel: [w352 FALSE] -> w344
        tunnel: [w350 FALSE] -> w342
        tunnel: w341 -> [w349 _]
        frame False {
          # "Data after first tick"
          n160 = case shown="真" "AI.B.DMA_ENA" {
            tunnel: w356 -> [w385 w393]
            tunnel: w355 -> [w373 _]
            tunnel: w351 -> [w376 _]
            tunnel: w354 -> [w372 _]
            tunnel: [w371 FALSE] -> w352
            tunnel: [FALSE w388] -> w350
            tunnel: w349 -> [_ w390]
            frame False {
              # "1 Sample"
              n161 = Add(x=w373, y=u8 8) -> (x+y=w383:u8)
              n162 = Select(t=w373, s=w372, f=w383) -> (s? t:f=w382:u8)
              n163 = feedback #18(fxp<+,4,4> 0.0 ("y")) -> (w377:fxp<+,4,4>)
              n164 = Increment(x=w377) -> (x+1=w379:fxp<+,4,4>)
              n165 = Greater?(x=w377, y=fxp<+,4,4> 11.0) -> (0:w371:bool)
              n166 = Select(t=w377, s=w371, f=w379) -> (s? t:f=w378:fxp<+,4,4>)
              n167 = Select(t=fxp<+,4,4> 0.0 ("y"), s=w376, f=w378) -> (s? t:f=w381:fxp<+,4,4>)
              n168 = feedback-in #18(w381) -> ()
              n169 = feedback #19(fxp<+/-,26,5>[] [0.0, 0.0, 0.0, 0.0, 0.0, 0.0, 0.0, 0.0, 0.0, 0.0, 0.0, 0.0] ("Array")) -> (w386:fxp<+/-,26,5>[])
              n170 = Replace Array Subset(array=w386, new element=w385, index=w382) -> (w358:fxp<+/-,26,5>[])
              n171 = feedback-in #19(w358) -> ()
              n172 = Index Array(array=w358) -> (element #1=→"AI.B_0.VAL":fxp<+/-,26,5>, element #2=→"AI.B_1.VAL":fxp<+/-,26,5>, element #3=→"AI.B_2.VAL":fxp<+/-,26,5>, element #4=→"AI.B_3.VAL":fxp<+/-,26,5>, element #5=→"AI.B_4.VAL":fxp<+/-,26,5>, element #6=→"AI.B_5.VAL":fxp<+/-,26,5>, element #7=→"AI.B_6.VAL":fxp<+/-,26,5>, element #8=→"AI.B_7.VAL":fxp<+/-,26,5>, element #9=→"AI.DIFF_B_0.VAL":fxp<+/-,26,5>, element #10=→"AI.DIFF_B_1.VAL":fxp<+/-,26,5>, element #11=→"AI.DIFF_B_2.VAL":fxp<+/-,26,5>, element #12=→"AI.DIFF_B_3.VAL":fxp<+/-,26,5>)  [unwired: 12 in]
            }
            frame True {
              # "N Sample"
              n173 = xnode ("FIFO Write")("元素"=w393, "超时"=0 ("Timeout")) -> ("超时？"=w389:bool)  [unwired: 1 in, 1 out]
              n174 = Or(x=w389, y=w390) -> (x .or. y?=w388:bool)
            }
          }
        }
        frame True {
          # "Data of first tick should not be acquired."
        }
      }
      "AI.B.VAL.RDY" <- w344
      "AI.B.DMA_FULL" <- w342
      n175 = feedback-in #17(w342) -> ()
    }
    n176 = node-c288(w316) -> ()
  }
  n177 = while {
    stop <- FALSE stop-if-true
    # "Push value buffer to A/AO0 pin"
    n178 = xnode ("FIFO Write")("超时"=-1 ("Timeout")) -> ("元素"=w401:fxp<+/-,20,5>)  [unwired: 1 in, 2 out]
    n179 = xnode "FPGA I/O Node"("ConnectorA/AO0"=w401) -> ()  [unwired: 1 in, 1 out]
  }
  n180 = while {
    stop <- FALSE stop-if-true
    # "AO 1 Sample Write Output"
    n181 = flat-sequence {
      frame #0 {
        # "Set the sample rate of the analog input \nsignal acquisition to 5 kHz."
        n182 = call "Loop Timer4"("Count(Ticks)"=u32 8000) -> ()  [unwired: 1 out]
      }
      frame #1 {
        n183 = local read "DATAGEN.ENA"() -> (w405:fxp<+,4,4>)
        n184 = feedback #20(FALSE) -> (w407:bool)
        n185 = case shown="真" "AO.SYS.GO" {
          tunnel: "AO.A_0.VAL" -> [_ w440]
          tunnel: "AO.B_0.VAL" -> [_ w439]
          tunnel: "AO.A_1.VAL" -> [_ w438]
          tunnel: "AO.B_1.VAL" -> [_ w437]
          tunnel: "AO.A.DMA_ENA" -> [_ w436]
          tunnel: [w416 w435] -> w408
          tunnel: w407 -> [w416 w434]
          tunnel: "AO.B.DMA_ENA" -> [_ w433]
          tunnel: w405 -> [_ w430]
          frame False {
          }
          frame True {
            n186 = Number To Boolean Array(number=w436) -> (Boolean array=w432:bool[])
            n187 = Number To Boolean Array(number=w430) -> (Boolean array=w429:bool[])
            n188 = Number To Boolean Array(number=w433) -> (Boolean array=w431:bool[])
            n189 = Index Array(array=w432) -> (element #1=w427:bool, element #2=w424:bool)  [unwired: 2 in]
            n190 = Index Array(array=w429) -> (element #1=w428:bool, element #2=w425:bool, element #3=w422:bool, element #4=w418:bool)  [unwired: 4 in]
            n191 = Index Array(array=w431) -> (element #1=w421:bool, element #2=w419:bool)  [unwired: 2 in]
            n192 = Or(x=w427, y=w428) -> (x .or. y?=w426:bool)
            n193 = Or(x=w424, y=w425) -> (x .or. y?=w423:bool)
            n194 = Or(x=w422, y=w421) -> (x .or. y?=w420:bool)
            n195 = Or(x=w418, y=w419) -> (x .or. y?=w417:bool)
            n196 = case shown="假" w426 {
              tunnel: w440 -> [w448 _]
              frame False {
                n197 = xnode ("FIFO Write")("元素"=w448, "超时"=-1 ("Timeout")) -> ()  [unwired: 1 in, 2 out]
              }
              frame True {
              }
            }
            n198 = case shown="假" w423 {
              tunnel: w438 -> [w445 _]
              frame False {
                n199 = xnode ("FIFO Write")("元素"=w445, "超时"=-1 ("Timeout")) -> ()  [unwired: 1 in, 2 out]
              }
              frame True {
              }
            }
            n200 = case shown="假" w420 {
              tunnel: w439 -> [w443 _]
              frame False {
                n201 = xnode ("FIFO Write")("元素"=w443, "超时"=-1 ("Timeout")) -> ()  [unwired: 1 in, 2 out]
              }
              frame True {
              }
            }
            n202 = case shown="假" w417 {
              tunnel: w437 -> [w441 _]
              frame False {
                n203 = xnode ("FIFO Write")("元素"=w441, "超时"=-1 ("Timeout")) -> ()  [unwired: 1 in, 2 out]
              }
              frame True {
              }
            }
            n204 = Not(x=w434) -> (.not. x?=w435:bool)
          }
        }
        "AO.SYS.STAT" <- w408
        n205 = feedback-in #20(w408) -> ()
      }
    }
  }
  n206 = node-c288() -> (w2:T2)  [unwired: 1 in]
  n207 = xnode "VI-Defined FIFO Configuration"() -> ()  [unwired: 1 out]
  n208 = xnode "VI-Defined Memory"() -> ()  [unwired: 1 out]
  n209 = xnode "VI-Defined Register"() -> ()  [unwired: 1 out]
  n210 = timed-loop {
    shift-right: [w499] -> _
    shift-left: _ -> [w497]
    timing: w2 -> [_]
    timing-out: [_] -> w1
    shift-right: [w465] -> _
    shift-left: _ -> [w462]
    shift-right: [w464] -> _
    shift-left: _ -> [w461]
    shift-right: [w463] -> _
    shift-left: _ -> [w460]
    stop <- FALSE stop-if-true
    # "Calculate the current DataGen output value on each tick by waveform frequency. It also provides the trigger to start all channels simultaneously"
    n211 = feedback #21() -> (w459:fxp<+,4,4>)  [unwired: 1 in]
    n212 = feedback-in #21("DATAGEN.ENA") -> ()
    n213 = Equal To 0?(x=w459) -> (x = 0?=w458:bool)
    n214 = Not Equal To 0?(x="DATAGEN.ENA") -> (x != 0?=w457:bool)
    n215 = Equal To 0?(x="DATAGEN.ENA") -> (x = 0?=w455:bool)
    n216 = And(x=w458, y=w457) -> (x .and. y?=w453:bool)
    n217 = Or(x=w453, y=w455) -> (x .or. y?=w454:bool)
    n218 = Number To Boolean Array(number="DATAGEN.A_0.FREQ_DIV") -> (Boolean array=w496:bool[])
    n219 = Number To Boolean Array(number="DATAGEN.A_1.FREQ_DIV") -> (Boolean array=w484:bool[])
    n220 = Number To Boolean Array(number="DATAGEN.B_0.FREQ_DIV") -> (Boolean array=w477:bool[])
    n221 = Number To Boolean Array(number="DATAGEN.B_1.FREQ_DIV") -> (Boolean array=w470:bool[])
    n222 = Select(t=u32 0, s=w454, f=w497) -> (s? t:f=w492:u32)
    n223 = Select(t=u32 0, s=w454, f=w462) -> (s? t:f=w487:u32)
    n224 = Select(t=u32 0, s=w454, f=w461) -> (s? t:f=w480:u32)
    n225 = Select(t=u32 0, s=w454, f=w460) -> (s? t:f=w473:u32)
    n226 = Boolean Array To Number(Boolean array=w496) -> (number=w495:u32)
    n227 = Boolean Array To Number(Boolean array=w484) -> (number=w485:u32)
    n228 = Boolean Array To Number(Boolean array=w477) -> (number=w478:u32)
    n229 = Boolean Array To Number(Boolean array=w470) -> (number=w471:u32)
    n230 = Add(x=w492, y=w495) -> (x+y=w499:u32)
    n231 = Add(x=w487, y=w485) -> (x+y=w465:u32)
    n232 = Add(x=w480, y=w478) -> (x+y=w464:u32)
    n233 = Add(x=w473, y=w471) -> (x+y=w463:u32)
    n234 = Logical Shift(y=i8 -19 ("accum shift"), x=w492) -> (x << y=w491:u32)
    n235 = Logical Shift(y=i8 -19 ("accum shift"), x=w487) -> (x << y=w488:u32)
    n236 = Logical Shift(y=i8 -19 ("accum shift"), x=w480) -> (x << y=w481:u32)
    n237 = Logical Shift(y=i8 -19 ("accum shift"), x=w473) -> (x << y=w474:u32)
    n238 = xnode ("Memory Read")("地址"=w491) -> ("数据"=w490:fxp<+/-,20,5>)  [unwired: 1 in, 1 out]
    n239 = xnode ("Memory Read")("地址"=w488) -> ("数据"=w489:fxp<+/-,20,5>)  [unwired: 1 in, 1 out]
    n240 = xnode ("Memory Read")("地址"=w481) -> ("数据"=w482:fxp<+/-,20,5>)  [unwired: 1 in, 1 out]
    n241 = xnode ("Memory Read")("地址"=w474) -> ("数据"=w475:fxp<+/-,20,5>)  [unwired: 1 in, 1 out]
    n242 = feedback-in #22(w490) -> ()
    n243 = feedback #22() -> (w452:fxp<+/-,20,5>)  [unwired: 1 in]
    n244 = feedback #23() -> (w451:fxp<+/-,20,5>)  [unwired: 1 in]
    n245 = feedback-in #23(w489) -> ()
    n246 = feedback #24() -> (w450:fxp<+/-,20,5>)  [unwired: 1 in]
    n247 = feedback-in #24(w482) -> ()
    n248 = feedback #25() -> (w449:fxp<+/-,20,5>)  [unwired: 1 in]
    n249 = feedback-in #25(w475) -> ()
    n250 = xnode ("Register Write")("数据"=w452) -> ()  [unwired: 1 in, 1 out]
    n251 = xnode ("Register Write")("数据"=w451) -> ()  [unwired: 1 in, 1 out]
    n252 = xnode ("Register Write")("数据"=w450) -> ()  [unwired: 1 in, 1 out]
    n253 = xnode ("Register Write")("数据"=w449) -> ()  [unwired: 1 in, 1 out]
  }
  n254 = xnode "VI-Defined FIFO Configuration"() -> ()  [unwired: 1 out]
  n255 = xnode "VI-Defined Memory"() -> ()  [unwired: 1 out]
  n256 = xnode "VI-Defined Register"() -> ()  [unwired: 1 out]
  n257 = xnode "VI-Defined FIFO Configuration"() -> ()  [unwired: 1 out]
  n258 = while {
    stop <- FALSE stop-if-true
    # "Push value buffer to A/AO1 pin"
    n259 = xnode ("FIFO Write")("超时"=-1 ("Timeout")) -> ("元素"=w504:fxp<+/-,20,5>)  [unwired: 1 in, 2 out]
    n260 = xnode "FPGA I/O Node"("ConnectorA/AO1"=w504) -> ()  [unwired: 1 in, 1 out]
  }
  n261 = xnode "VI-Defined FIFO Configuration"() -> ()  [unwired: 1 out]
  n262 = xnode "VI-Defined Memory"() -> ()  [unwired: 1 out]
  n263 = xnode "VI-Defined Register"() -> ()  [unwired: 1 out]
  n264 = xnode "VI-Defined Memory"() -> ()  [unwired: 1 out]
  n265 = xnode "VI-Defined Register"() -> ()  [unwired: 1 out]
  n266 = while {
    stop <- FALSE stop-if-true
    # "Push value buffer to B/AO0 pin"
    n267 = xnode ("FIFO Write")("超时"=-1 ("Timeout")) -> ("元素"=w507:fxp<+/-,20,5>)  [unwired: 1 in, 2 out]
    n268 = xnode "FPGA I/O Node"("ConnectorB/AO0"=w507) -> ()  [unwired: 1 in, 1 out]
  }
  n269 = node-c288(w1) -> ()
  n270 = Generate Occurrence() -> (w9:refnum<k4>)
  n271 = while {
    stop <- FALSE stop-if-true
    # "Push value buffer to B/AO1 pin"
    n272 = xnode ("FIFO Write")("超时"=-1 ("Timeout")) -> ("元素"=w510:fxp<+/-,20,5>)  [unwired: 1 in, 2 out]
    n273 = xnode "FPGA I/O Node"("ConnectorB/AO1"=w510) -> ()  [unwired: 1 in, 1 out]
  }
  n274 = node-c288() -> (w11:T2)  [unwired: 1 in]
  n275 = while {
    shift-right: [w515] -> _
    shift-left: w6 -> [w516]
    stop <- FALSE stop-if-true
    # "Update the full waveform in the DataGen buffer for A/AO0"
    n276 = xnode ("FIFO Read")("超时"=-1 ("Timeout")) -> ("元素"=w517:i32, "超时？"=w512:bool)  [unwired: 1 in, 1 out]
    n277 = node-c288() -> (w514:T2)  [unwired: 1 in]
    n278 = timed-loop {
      timing: w514 -> [_]
      timing-out: [_] -> w513
      tunnel: w517 -> [w528]
      tunnel: w512 -> [w526]
      shift-right: [w523] -> w515
      shift-left: w516 -> [w527]
      stop <- TRUE stop-if-true
      n279 = case shown="假" w526 {
        tunnel: w528 -> [w533 _]
        tunnel: w527 -> [w534 w536]
        tunnel: [w535 w536] -> w522
        frame False {
          n280 = Number To Boolean Array(number=w533) -> (Boolean array=w531:bool[])
          n281 = Array Subset(array=w531, index=12) -> (w532:bool[])  [unwired: 1 in]
          n282 = Boolean Array To Number(Boolean array=w532) -> (number=w529:fxp<+/-,20,5>)
          n283 = Increment(x=w534) -> (x+1=w535:u32)
          n284 = xnode ("Memory Write")("地址"=w534, "数据"=w529) -> ()  [unwired: 1 in, 1 out]
        }
        frame True {
        }
      }
      n285 = Less?(x=w522, y=u32 8192) -> (x < y?=w524:bool)
      n286 = Select(t=w522, s=w524, f=u32 0 ("Address")) -> (s? t:f=w523:u32)
    }
    n287 = node-c288(w513) -> ()
  }
  n288 = while {
    stop <- FALSE stop-if-true
    # "Feed the A/AO0 value buffer from DataGen"
    n289 = flat-sequence {
      frame #0 {
        n290 = call "Loop Timer7"("Count(Ticks)"="DATAGEN.A_0.CNTR") -> ()  [unwired: 1 out]
      }
      frame #1 {
        n291 = local read "DATAGEN.ENA"() -> (w543:fxp<+,4,4>)
        n292 = Number To Boolean Array(number=w543) -> (Boolean array=w544:bool[])
        n293 = Index Array(array=w544) -> (element=w545:bool)  [unwired: 1 in]
        n294 = case shown="真" w545 {
          frame False {
          }
          frame True {
            n295 = xnode ("Register Read")() -> ("数据"=w547:fxp<+/-,20,5>)  [unwired: 1 in, 1 out]
            n296 = xnode ("FIFO Write")("元素"=w547, "超时"=-1 ("Timeout")) -> ()  [unwired: 1 in, 2 out]
          }
        }
      }
    }
  }
  n297 = while {
    tunnel: w9 -> [w548]
    stop <- FALSE stop-if-true
    # "A/AO N Samples Write Output"
    n298 = flat-sequence {
      tunnel: w548 -> [w550]
      frame #0 {
        n299 = case shown="真" "AO.A.SYNC" {
          tunnel: w550 -> [_ w553]
          frame False {
          }
          frame True {
            n300 = Wait on Occurrence(2:w553, 3:10000 ("ms timeout (-1)")) -> ()  [unwired: 1 in, 1 out]
          }
        }
        n301 = call "Loop Timer2"("Count(Ticks)"="AO.A.DMA_CNTR") -> ()  [unwired: 1 out]
      }
      frame #1 {
        n302 = node-c288() -> (w562:T2)  [unwired: 1 in]
        n303 = timed-loop {
          timing: w562 -> [_]
          timing-out: [_] -> w561
          tunnel: [w593] -> w560
          shift-right: [w590] -> w559
          shift-left: _ -> [w592]
          shift-right: [w591] -> w558
          shift-left: _ -> [w589]
          tunnel: [w575] -> w556
          tunnel: [w572] -> w555
          i -> [w597]
          stop <- w598 stop-if-true
          # ">>AO1 Cache Data>>"
          # ">>AO0 Cache Data>>"
          n304 = local read "DATAGEN.ENA"() -> (w578:fxp<+,4,4>)
          n305 = local read "AO.A.DMA_ENA"() -> (w582:fxp<+,2,2>)
          n306 = Number To Boolean Array(number=w582) -> (Boolean array=w599:bool[])
          n307 = Number To Boolean Array(number=w578) -> (Boolean array=w579:bool[])
          n308 = case shown="默认" w582 {
            tunnel: [TRUE ("Timed Out?") w606] -> w588
            tunnel: [0 ("Element") w605] -> w584
            frame 0 {
            }
            frame Default {
              n309 = xnode ("FIFO Read")("超时"=u16 0 ("Timeout")) -> ("元素"=w605:fxp<+/-,20,5>, "超时？"=w606:bool)  [unwired: 1 in, 1 out]
            }
          }
          "AO.A.DMA_IDL" <- w588
          n310 = Index Array(array=w599) -> (element #1=w595:bool, element #2=w594:bool)  [unwired: 2 in]
          n311 = Index Array(array=w579) -> (element #1=w580:bool, element #2=w581:bool)  [unwired: 2 in]
          n312 = Boolean To (0,1)(Boolean=w595) -> (0, 1=w600:i16)
          n313 = Boolean To (0,1)(Boolean=w594) -> (0, 1=w601:i16)
          n314 = Not(x=w581) -> (.not. x?=w573:bool)
          n315 = Not(x=w580) -> (.not. x?=w576:bool)
          n316 = Add(x=w600, y=w601) -> (x+y=w596:i16)
          n317 = Number To Boolean Array(number=w584) -> (Boolean array=w586:bool[])
          n318 = Increment(x=w597) -> (x+1=w602:i32)
          n319 = Less Or Equal?(x=w596, y=w602) -> (x <= y?=w598:bool)
          n320 = Array Subset(array=w586, index=12) -> (w585:bool[])  [unwired: 1 in]
          n321 = Not(x=w588) -> (.not. x?=w593:bool)
          n322 = Boolean Array To Number(Boolean array=w585) -> (number=w583:fxp<+/-,20,5>)
          n323 = case shown="1" w596 {
            tunnel: [w609 w613 w623] -> w590
            tunnel: w583 -> [_ w614 w622]
            tunnel: w595 -> [_ w615 _]
            tunnel: w597 -> [_ _ w625]
            tunnel: w592 -> [w609 w611 w621]
            tunnel: [w608 w612 w624] -> w591
            tunnel: w589 -> [w608 w610 w620]
            frame 0, Default {
              # "No N sample channel"
            }
            frame 1 {
              # "1 N Sample channel"
              n324 = case shown="假" w615 {
                tunnel: w614 -> [w617 w619]
                tunnel: [w616 w619] -> w613
                tunnel: [w617 w618] -> w612
                tunnel: w611 -> [w616 _]
                tunnel: w610 -> [_ w618]
                frame False {
                  # "AO 1"
                }
                frame True {
                  # "AO 0"
                }
              }
            }
            frame 2 {
              # "2 N Sample channels"
              n325 = case shown="0, 默认" w625 {
                tunnel: [w627 w628] -> w623
                tunnel: [w626 w629] -> w624
                tunnel: w622 -> [w627 w629]
                tunnel: w621 -> [_ w628]
                tunnel: w620 -> [w626 _]
                frame 0, Default {
                  # "AO 0"
                }
                frame 1 {
                  # "AO 1"
                }
              }
            }
          }
          n326 = And(x=w595, y=w593) -> (x .and. y?=w577:bool)
          n327 = And(x=w593, y=w594) -> (x .and. y?=w574:bool)
          n328 = And(x=w577, y=w576) -> (x .and. y?=w575:bool)
          n329 = And(x=w574, y=w573) -> (x .and. y?=w572:bool)
        }
        n330 = global read "ELVIS III Global.vi" "AO.A.DMA_IRQ_NO"() -> (w557:u8)
        n331 = call "Falling Edge Trigger.vi"("Signal"=w560) -> ("Trigger?"=w566:bool)
        n332 = feedback #26(FALSE ("Timed Out?")) -> (w563:bool)
        n333 = Or(x=w566, y=w563) -> (x .or. y?=w567:bool)
        n334 = case shown="真" w567 {
          selector: w567 -> [w634 _]
          tunnel: [w634 w636] -> w565
          tunnel: w557 -> [_ w635]
          frame False {
          }
          frame True {
            # "Send wirte finish IRQ"
            n335 = xnode ("FIFO Write")("元素"=w635, "超时"=0 ("Timeout")) -> ("超时？"=w636:bool)  [unwired: 1 in, 1 out]
          }
        }
        n336 = feedback-in #26(w565) -> ()
        n337 = node-c288(w561) -> ()
        n338 = case shown="真" w556 {
          tunnel: w559 -> [_ w570]
          frame False {
            # "Timeout or channel not selected"
          }
          frame True {
            n339 = xnode ("FIFO Write")("元素"=w570, "超时"=-1 ("Timeout")) -> ()  [unwired: 1 in, 2 out]
          }
        }
        n340 = case shown="真" w555 {
          tunnel: w558 -> [_ w569]
          frame False {
            # "Timeout or channel not selected"
          }
          frame True {
            n341 = xnode ("FIFO Write")("元素"=w569, "超时"=-1 ("Timeout")) -> ()  [unwired: 1 in, 2 out]
          }
        }
      }
    }
  }
  n342 = timed-loop {
    tunnel: w9 -> [w642]
    timing: w11 -> [_]
    timing-out: [_] -> w10
    stop <- FALSE stop-if-true
    n343 = xnode ("FIFO Write")() -> ("待读取元素数量"=→"AO.A.ELE_NUM":u32)  [unwired: 1 in, 1 out]
    n344 = xnode ("FIFO Write")() -> ("待读取元素数量"=→"AO.B.ELE_NUM":u32)  [unwired: 1 in, 1 out]
    n345 = case shown="真" "AO.SYNC" {
      tunnel: w642 -> [_ w643]
      frame False {
      }
      frame True {
        n346 = Set Occurrence(w643) -> ()
      }
    }
  }
  n347 = node-c288(w10) -> ()
  n348 = while {
    shift-right: [w648] -> _
    shift-left: w5 -> [w650]
    stop <- FALSE stop-if-true
    # "Update the full waveform in the DataGen buffer for A/AO1"
    n349 = xnode ("FIFO Read")("超时"=-1 ("Timeout")) -> ("元素"=w651:i32, "超时？"=w649:bool)  [unwired: 1 in, 1 out]
    n350 = node-c288() -> (w647:T2)  [unwired: 1 in]
    n351 = timed-loop {
      timing: w647 -> [_]
      timing-out: [_] -> w646
      tunnel: w651 -> [w662]
      tunnel: w649 -> [w660]
      shift-right: [w657] -> w648
      shift-left: w650 -> [w661]
      stop <- TRUE stop-if-true
      n352 = case shown="假" w660 {
        tunnel: w662 -> [w667 _]
        tunnel: w661 -> [w668 w670]
        tunnel: [w669 w670] -> w656
        frame False {
          n353 = Number To Boolean Array(number=w667) -> (Boolean array=w665:bool[])
          n354 = Array Subset(array=w665, index=12) -> (w664:bool[])  [unwired: 1 in]
          n355 = Boolean Array To Number(Boolean array=w664) -> (number=w663:fxp<+/-,20,5>)
          n356 = Increment(x=w668) -> (x+1=w669:u32)
          n357 = xnode ("Memory Write")("地址"=w668, "数据"=w663) -> ()  [unwired: 1 in, 1 out]
        }
        frame True {
        }
      }
      n358 = Less?(x=w656, y=u32 8192) -> (x < y?=w658:bool)
      n359 = Select(t=w656, s=w658, f=u32 0 ("Address")) -> (s? t:f=w657:u32)
    }
    n360 = node-c288(w646) -> ()
  }
  n361 = while {
    stop <- FALSE stop-if-true
    # "Feed the A/AO1 value buffer from DataGen"
    n362 = flat-sequence {
      frame #0 {
        n363 = call "Loop Timer8"("Count(Ticks)"="DATAGEN.A_1.CNTR") -> ()  [unwired: 1 out]
      }
      frame #1 {
        n364 = local read "DATAGEN.ENA"() -> (w679:fxp<+,4,4>)
        n365 = Number To Boolean Array(number=w679) -> (Boolean array=w680:bool[])
        n366 = Index Array(array=w680, index=1) -> (element=w677:bool)
        n367 = case shown="真" w677 {
          frame False {
          }
          frame True {
            n368 = xnode ("Register Read")() -> ("数据"=w682:fxp<+/-,20,5>)  [unwired: 1 in, 1 out]
            n369 = xnode ("FIFO Write")("元素"=w682, "超时"=-1 ("Timeout")) -> ()  [unwired: 1 in, 2 out]
          }
        }
      }
    }
  }
  n370 = while {
    tunnel: w9 -> [w683]
    stop <- FALSE stop-if-true
    # "B/AO N Samples Write Output"
    n371 = flat-sequence {
      tunnel: w683 -> [w685]
      frame #0 {
        n372 = case shown="真" "AO.B.SYNC" {
          tunnel: w685 -> [_ w688]
          frame False {
          }
          frame True {
            n373 = Wait on Occurrence(2:w688, 3:10000 ("ms timeout (-1)")) -> ()  [unwired: 1 in, 1 out]
          }
        }
        n374 = call "Loop Timer3"("Count(Ticks)"="AO.B.DMA_CNTR") -> ()  [unwired: 1 out]
      }
      frame #1 {
        n375 = node-c288() -> (w697:T2)  [unwired: 1 in]
        n376 = timed-loop {
          timing: w697 -> [_]
          timing-out: [_] -> w696
          tunnel: [w730] -> w695
          shift-right: [w727] -> w694
          shift-left: _ -> [w729]
          shift-right: [w728] -> w693
          shift-left: _ -> [w726]
          tunnel: [w710] -> w691
          tunnel: [w707] -> w690
          i -> [w734]
          stop <- w735 stop-if-true
          # ">>AO1 Cache Data>>"
          # ">>AO0 Cache Data>>"
          n377 = local read "AO.B.DMA_ENA"() -> (w719:fxp<+,2,2>)
          n378 = local read "DATAGEN.ENA"() -> (w718:fxp<+,4,4>)
          n379 = Number To Boolean Array(number=w719) -> (Boolean array=w736:bool[])
          n380 = Number To Boolean Array(number=w718) -> (Boolean array=w717:bool[])
          n381 = case shown="默认" w719 {
            tunnel: [TRUE ("Timed Out?") w743] -> w725
            tunnel: [0 ("Element") w742] -> w721
            frame 0 {
            }
            frame Default {
              n382 = xnode ("FIFO Read")("超时"=u16 0 ("Timeout")) -> ("元素"=w742:fxp<+/-,20,5>, "超时？"=w743:bool)  [unwired: 1 in, 1 out]
            }
          }
          "AO.B.DMA_IDL" <- w725
          n383 = Index Array(array=w736) -> (element #1=w732:bool, element #2=w731:bool)  [unwired: 2 in]
          n384 = Index Array(array=w717, index #1=2 ("index"), index #2=3 ("index")) -> (element #1=w714:bool, element #2=w713:bool)
          n385 = Boolean To (0,1)(Boolean=w732) -> (0, 1=w737:i16)
          n386 = Boolean To (0,1)(Boolean=w731) -> (0, 1=w738:i16)
          n387 = Not(x=w714) -> (.not. x?=w711:bool)
          n388 = Not(x=w713) -> (.not. x?=w708:bool)
          n389 = Add(x=w737, y=w738) -> (x+y=w733:i16)
          n390 = Increment(x=w734) -> (x+1=w739:i32)
          n391 = Number To Boolean Array(number=w721) -> (Boolean array=w723:bool[])
          n392 = Less Or Equal?(x=w733, y=w739) -> (x <= y?=w735:bool)
          n393 = Not(x=w725) -> (.not. x?=w730:bool)
          n394 = Array Subset(array=w723, index=12) -> (w722:bool[])  [unwired: 1 in]
          n395 = Boolean Array To Number(Boolean array=w722) -> (number=w720:fxp<+/-,20,5>)
          n396 = case shown="0, 默认" w733 {
            tunnel: [w746 w750 w760] -> w727
            tunnel: w720 -> [_ w751 w759]
            tunnel: w732 -> [_ w752 _]
            tunnel: w734 -> [_ _ w762]
            tunnel: w729 -> [w746 w748 w758]
            tunnel: [w745 w749 w761] -> w728
            tunnel: w726 -> [w745 w747 w757]
            frame 0, Default {
              # "No N sample channel"
            }
            frame 1 {
              # "1 N Sample channel"
              n397 = case shown="真" w752 {
                tunnel: w751 -> [w754 w756]
                tunnel: [w753 w756] -> w750
                tunnel: [w754 w755] -> w749
                tunnel: w748 -> [w753 _]
                tunnel: w747 -> [_ w755]
                frame False {
                  # "AO 1"
                }
                frame True {
                  # "AO 0"
                }
              }
            }
            frame 2 {
              # "2 N Sample channels"
              n398 = case shown="1" w762 {
                tunnel: [w764 w765] -> w760
                tunnel: [w763 w766] -> w761
                tunnel: w759 -> [w764 w766]
                tunnel: w758 -> [_ w765]
                tunnel: w757 -> [w763 _]
                frame 0, Default {
                  # "AO 0"
                }
                frame 1 {
                  # "AO 1"
                }
              }
            }
          }
          n399 = And(x=w732, y=w730) -> (x .and. y?=w712:bool)
          n400 = And(x=w730, y=w731) -> (x .and. y?=w709:bool)
          n401 = And(x=w712, y=w711) -> (x .and. y?=w710:bool)
          n402 = And(x=w709, y=w708) -> (x .and. y?=w707:bool)
        }
        n403 = global read "ELVIS III Global.vi" "AO.B.DMA_IRQ_NO"() -> (w692:u8)
        n404 = call "Falling Edge Trigger.vi"("Signal"=w695) -> ("Trigger?"=w701:bool)
        n405 = feedback #27(FALSE ("Timed Out?")) -> (w698:bool)
        n406 = Or(x=w701, y=w698) -> (x .or. y?=w702:bool)
        n407 = case shown="真" w702 {
          selector: w702 -> [w771 _]
          tunnel: [w771 w773] -> w700
          tunnel: w692 -> [_ w772]
          frame False {
          }
          frame True {
            # "Send wirte finish IRQ"
            n408 = xnode ("FIFO Write")("元素"=w772, "超时"=0 ("Timeout")) -> ("超时？"=w773:bool)  [unwired: 1 in, 1 out]
          }
        }
        n409 = feedback-in #27(w700) -> ()
        n410 = node-c288(w696) -> ()
        n411 = case shown="真" w691 {
          tunnel: w694 -> [_ w706]
          frame False {
            # "Timeout or channel not selected"
          }
          frame True {
            n412 = xnode ("FIFO Write")("元素"=w706, "超时"=-1 ("Timeout")) -> ()  [unwired: 1 in, 2 out]
          }
        }
        n413 = case shown="真" w690 {
          tunnel: w693 -> [_ w704]
          frame False {
            # "Timeout or channel not selected"
          }
          frame True {
            n414 = xnode ("FIFO Write")("元素"=w704, "超时"=-1 ("Timeout")) -> ()  [unwired: 1 in, 2 out]
          }
        }
      }
    }
  }
  n415 = while {
    shift-right: [w777] -> _
    shift-left: w4 -> [w779]
    stop <- FALSE stop-if-true
    # "Update the full waveform in the DataGen buffer for B/AO0"
    n416 = xnode ("FIFO Read")("超时"=-1 ("Timeout")) -> ("元素"=w780:i32, "超时？"=w778:bool)  [unwired: 1 in, 1 out]
    n417 = node-c288() -> (w776:T2)  [unwired: 1 in]
    n418 = timed-loop {
      timing: w776 -> [_]
      timing-out: [_] -> w775
      tunnel: w780 -> [w791]
      tunnel: w778 -> [w789]
      shift-right: [w786] -> w777
      shift-left: w779 -> [w790]
      stop <- TRUE stop-if-true
      n419 = case shown="假" w789 {
        tunnel: w791 -> [w796 _]
        tunnel: w790 -> [w797 w799]
        tunnel: [w798 w799] -> w785
        frame False {
          n420 = Number To Boolean Array(number=w796) -> (Boolean array=w794:bool[])
          n421 = Array Subset(array=w794, index=12) -> (w793:bool[])  [unwired: 1 in]
          n422 = Boolean Array To Number(Boolean array=w793) -> (number=w792:fxp<+/-,20,5>)
          n423 = xnode ("Memory Write")("地址"=w797, "数据"=w792) -> ()  [unwired: 1 in, 1 out]
          n424 = Increment(x=w797) -> (x+1=w798:u32)
        }
        frame True {
        }
      }
      n425 = Less?(x=w785, y=u32 8192) -> (x < y?=w787:bool)
      n426 = Select(t=w785, s=w787, f=u32 0 ("Address")) -> (s? t:f=w786:u32)
    }
    n427 = node-c288(w775) -> ()
  }
  n428 = while {
    stop <- FALSE stop-if-true
    # "Feed the B/AO0 value buffer from DataGen"
    n429 = flat-sequence {
      frame #0 {
        n430 = call "Loop Timer9"("Count(Ticks)"="DATAGEN.B_0.CNTR") -> ()  [unwired: 1 out]
      }
      frame #1 {
        n431 = local read "DATAGEN.ENA"() -> (w808:fxp<+,4,4>)
        n432 = Number To Boolean Array(number=w808) -> (Boolean array=w809:bool[])
        n433 = Index Array(array=w809, index=2) -> (element=w806:bool)
        n434 = case shown="真" w806 {
          frame False {
          }
          frame True {
            n435 = xnode ("Register Read")() -> ("数据"=w811:fxp<+/-,20,5>)  [unwired: 1 in, 1 out]
            n436 = xnode ("FIFO Write")("元素"=w811, "超时"=-1 ("Timeout")) -> ()  [unwired: 1 in, 2 out]
          }
        }
      }
    }
  }
  n437 = while {
    shift-right: [w814] -> _
    shift-left: w3 -> [w816]
    stop <- FALSE stop-if-true
    # "Update the full waveform in the DataGen buffer for B/AO1"
    n438 = xnode ("FIFO Read")("超时"=-1 ("Timeout")) -> ("元素"=w817:i32, "超时？"=w815:bool)  [unwired: 1 in, 1 out]
    n439 = node-c288() -> (w813:T2)  [unwired: 1 in]
    n440 = timed-loop {
      timing: w813 -> [_]
      timing-out: [_] -> w812
      tunnel: w817 -> [w828]
      tunnel: w815 -> [w826]
      shift-right: [w823] -> w814
      shift-left: w816 -> [w827]
      stop <- TRUE stop-if-true
      n441 = case shown="假" w826 {
        tunnel: w828 -> [w833 _]
        tunnel: w827 -> [w834 w836]
        tunnel: [w835 w836] -> w822
        frame False {
          n442 = Number To Boolean Array(number=w833) -> (Boolean array=w831:bool[])
          n443 = Array Subset(array=w831, index=12) -> (w830:bool[])  [unwired: 1 in]
          n444 = Boolean Array To Number(Boolean array=w830) -> (number=w829:fxp<+/-,20,5>)
          n445 = Increment(x=w834) -> (x+1=w835:u32)
          n446 = xnode ("Memory Write")("地址"=w834, "数据"=w829) -> ()  [unwired: 1 in, 1 out]
        }
        frame True {
        }
      }
      n447 = Less?(x=w822, y=u32 8192) -> (x < y?=w824:bool)
      n448 = Select(t=w822, s=w824, f=u32 0 ("Address")) -> (s? t:f=w823:u32)
    }
    n449 = node-c288(w812) -> ()
  }
  n450 = while {
    stop <- FALSE stop-if-true
    # "Feed the B/AO1 value buffer from DataGen"
    n451 = flat-sequence {
      frame #0 {
        n452 = call "Loop Timer10"("Count(Ticks)"="DATAGEN.B_1.CNTR") -> ()  [unwired: 1 out]
      }
      frame #1 {
        n453 = local read "DATAGEN.ENA"() -> (w845:fxp<+,4,4>)
        n454 = Number To Boolean Array(number=w845) -> (Boolean array=w846:bool[])
        n455 = Index Array(array=w846, index=3) -> (element=w844:bool)
        n456 = case shown="真" w844 {
          frame False {
          }
          frame True {
            n457 = xnode ("Register Read")() -> ("数据"=w848:fxp<+/-,20,5>)  [unwired: 1 in, 1 out]
            n458 = xnode ("FIFO Write")("元素"=w848, "超时"=-1 ("Timeout")) -> ()  [unwired: 1 in, 2 out]
          }
        }
      }
    }
  }
  n459 = xnode "VI-Defined FIFO Configuration"() -> ("FIFO输出"=w15:refnum<k21>)
  n460 = node-c288() -> (w17:T2)  [unwired: 1 in]
  n461 = timed-loop {
    timing: w17 -> [_]
    timing-out: [_] -> w16
    tunnel: w15 -> [w851]
    stop <- _ stop-if-true
    # "Onboard I/O"
    n462 = xnode "FPGA I/O Node"() -> ("Button0"=w855:bool)  [unwired: 1 in, 1 out]
    n463 = Number To Boolean Array(number="DO.LED3:0") -> (Boolean array=w860:bool[])
    n464 = Build Array(w855) -> (w863:bool[])
    n465 = Index Array(array=w860) -> (element #1=w859:bool, element #2=w858:bool, element #3=w857:bool, element #4=w856:bool)  [unwired: 4 in]
    n466 = call "DIO IRQ 1-bit.vi"("IRQ.NO"="IRQ.DI_BTN.NO", "IRQ.CNT"="IRQ.DI_BTN.CNT", "FIFO in"=w851, "IRQ.FALL"="IRQ.DI_BTN.FALL", "IRQ.RISE"="IRQ.DI_BTN.RISE", "IRQ.ENA"="IRQ.DI_BTN.ENA", "DIO"=w855) -> ()  [unwired: 5 in]
    n467 = Boolean Array To Number(Boolean array=w863) -> (number=→"DI.BTN":u8)
    n468 = xnode "FPGA I/O Node"("LED0"=w859, "LED1"=w858, "LED2"=w857, "LED3"=w856) -> ()  [unwired: 4 in, 4 out]
  }
  n469 = while {
    stop <- FALSE stop-if-true
    # "Button SCTL Interrupt Buffer"
    n470 = feedback #28(u8 0 ("Element")) -> (w868:u8)
    n471 = feedback #29(FALSE ("Timed Out?")) -> (w872:bool)
    n472 = case shown="假" w872 {
      tunnel: [w874 w876] -> w869
      tunnel: w868 -> [_ w876]
      frame False {
        n473 = xnode ("FIFO Method Node")("超时"=-1 ("Timeout")) -> ("元素"=w874:u8)  [unwired: 1 in, 2 out]
      }
      frame True {
      }
    }
    n474 = feedback-in #28(w869) -> ()
    n475 = xnode ("FIFO Method Node")("元素"=w869, "超时"=0 ("Timeout")) -> ("超时？"=w870:bool)  [unwired: 1 in, 1 out]
    n476 = feedback-in #29(w870) -> ()
  }
  n477 = node-c288(w16) -> ()
  n478 = node-c288() -> (w22:T2)  [unwired: 1 in]
  n479 = xnode "VI-Defined FIFO Configuration"() -> ()  [unwired: 1 out]
  n480 = timed-loop {
    timing: w22 -> [_]
    timing-out: [_] -> w21
    stop <- _ stop-if-true
    w885 = u16 5 ("Debounce Ticks")
    w920 = u8 0
    w981 = T5 {"ENC.CNFG"=0, "ENC.CNTR"=0, "ENC.STAT"=0}  # Encoder.GROUP
    w972 = T6 {"PWM.0.CS"=0, "PWM.0.CNFG"=0, "PWM.0.CMP"=0, "PWM.0.MAX"=0, "PWM.0.CNTR"=0, "PWM.1.CS"=0, "PWM.1.CNFG"=0, "PWM.1.CMP"=0, "PWM.1.MAX"=0, "PWM.1.CNTR"=0}  # PWM.GROUP
    w1010 = T5 {"ENC.CNFG"=0, "ENC.CNTR"=0, "ENC.STAT"=0}  # Encoder.GROUP
    w1019 = T6 {"PWM.0.CS"=0, "PWM.0.CNFG"=0, "PWM.0.CMP"=0, "PWM.0.MAX"=0, "PWM.0.CNTR"=0, "PWM.1.CS"=0, "PWM.1.CNFG"=0, "PWM.1.CMP"=0, "PWM.1.MAX"=0, "PWM.1.CNTR"=0}  # PWM.GROUP
    w1030 = T7 {"I2C.GO"=FALSE, "I2C.CNFG"=1, "I2C.DATO"=0, "I2C.DATI"=0, "I2C.ADDR"=0, "I2C.CNTR"=213, "I2C.CNTL"=0, "I2C.STAT"=0}  # I2C.GROUP
    w1041 = T5 {"ENC.CNFG"=0, "ENC.CNTR"=0, "ENC.STAT"=0}  # Encoder.GROUP
    w1032 = T6 {"PWM.0.CS"=0, "PWM.0.CNFG"=0, "PWM.0.CMP"=0, "PWM.0.MAX"=0, "PWM.0.CNTR"=0, "PWM.1.CS"=0, "PWM.1.CNFG"=0, "PWM.1.CMP"=0, "PWM.1.MAX"=0, "PWM.1.CNTR"=0}  # PWM.GROUP
    w1063 = T5 {"ENC.CNFG"=0, "ENC.CNTR"=0, "ENC.STAT"=0}  # Encoder.GROUP
    w1072 = T6 {"PWM.0.CS"=0, "PWM.0.CNFG"=0, "PWM.0.CMP"=0, "PWM.0.MAX"=0, "PWM.0.CNTR"=0, "PWM.1.CS"=0, "PWM.1.CNFG"=0, "PWM.1.CMP"=0, "PWM.1.MAX"=0, "PWM.1.CNTR"=0}  # PWM.GROUP
    w1085 = T5 {"ENC.CNFG"=0, "ENC.CNTR"=0, "ENC.STAT"=0}  # Encoder.GROUP
    w1076 = T6 {"PWM.0.CS"=0, "PWM.0.CNFG"=0, "PWM.0.CMP"=0, "PWM.0.MAX"=0, "PWM.0.CNTR"=0, "PWM.1.CS"=0, "PWM.1.CNFG"=0, "PWM.1.CMP"=0, "PWM.1.MAX"=0, "PWM.1.CNTR"=0}  # PWM.GROUP
    w1109 = T5 {"ENC.CNFG"=0, "ENC.CNTR"=0, "ENC.STAT"=0}  # Encoder.GROUP
    w1100 = T6 {"PWM.0.CS"=0, "PWM.0.CNFG"=0, "PWM.0.CMP"=0, "PWM.0.MAX"=0, "PWM.0.CNTR"=0, "PWM.1.CS"=0, "PWM.1.CNFG"=0, "PWM.1.CMP"=0, "PWM.1.MAX"=0, "PWM.1.CNTR"=0}  # PWM.GROUP
    w1125 = T8 {"SPI.STAT"=0, "SPI.GO"=FALSE, "SPI.CNT"=19, "SPI.CNFG"=112, "SPI.DATI"=0, "SPI.DATO"=0}  # SPI.GROUP
    w954 = T5 {"ENC.CNFG"=0, "ENC.CNTR"=0, "ENC.STAT"=0}  # Encoder.GROUP
    w955 = T6 {"PWM.0.CS"=0, "PWM.0.CNFG"=0, "PWM.0.CMP"=0, "PWM.0.MAX"=0, "PWM.0.CNTR"=0, "PWM.1.CS"=0, "PWM.1.CNFG"=0, "PWM.1.CMP"=0, "PWM.1.MAX"=0, "PWM.1.CNTR"=0}  # PWM.GROUP
    w1163 = T5 {"ENC.CNFG"=0, "ENC.CNTR"=0, "ENC.STAT"=0}  # Encoder.GROUP
    w1162 = T6 {"PWM.0.CS"=0, "PWM.0.CNFG"=0, "PWM.0.CMP"=0, "PWM.0.MAX"=0, "PWM.0.CNTR"=0, "PWM.1.CS"=0, "PWM.1.CNFG"=0, "PWM.1.CMP"=0, "PWM.1.MAX"=0, "PWM.1.CNTR"=0}  # PWM.GROUP
    w1184 = T5 {"ENC.CNFG"=0, "ENC.CNTR"=0, "ENC.STAT"=0}  # Encoder.GROUP
    w1193 = T6 {"PWM.0.CS"=0, "PWM.0.CNFG"=0, "PWM.0.CMP"=0, "PWM.0.MAX"=0, "PWM.0.CNTR"=0, "PWM.1.CS"=0, "PWM.1.CNFG"=0, "PWM.1.CMP"=0, "PWM.1.MAX"=0, "PWM.1.CNTR"=0}  # PWM.GROUP
    # "DIO/UART Error Handling"
    # "DIO/PWM/Encoder"
    # "DIO/PWM/Encoder"
    # "DIO/PWM/Encoder/I2C"
    # "DIO/PWM/Encoder"
    # "DIO/PWM/Encoder"
    # ">>A.DIO_19:0.OUT>>"
    # "DIO/PWM/Encoder"
    # "DIO/PWM/Encoder/SPI"
    # "DIO/PWM/Encoder"
    # "DIO/PWM/Encoder"
    # "TODO:\nAdd DIO INT here."
    # "Write DIO"
    # "Read DIO"
    # "DIO Bank A"
    n481 = call "DIO Write Bank.vi"("DIO.19:0.OUT"="DIO.A_19:0.OUT", "DO.DMA_CNTR"="DO.A.DMA_CNTR", "DO.DMA_ENA"="DO.A.DMA_ENA", "DMA FIFO IN"=refnum<k21> "DO.A.DMA" ("DMA FIFO In")) -> ("DO.DMA_IDL"=w1197:bool, "DATA OUT"=w1194:fxp<+,20,20>)  [unwired: 6 in]
    "DO.A.DMA_IDL" <- w1197
    n482 = call "Split Bank DIO.vi"("IN 19:0"=w1194) -> ("OUT 1:0"=w1182:fxp<+,2,2>, "OUT 3:2"=w1146:fxp<+,2,2>, "OUT 7:4"=w1141:fxp<+,4,4>, "OUT 9:8"=w1099:fxp<+,2,2>, "OUT 11:10"=w1075:fxp<+,2,2>, "OUT 13:12"=w998:fxp<+,2,2>, "OUT 19:18"=w968:fxp<+,2,2>, "OUT 17:16"=w971:fxp<+,2,2>, "OUT 15:14"=w996:fxp<+,2,2>)  [unwired: 6 in]
    n483 = call "Split Bank DIO.vi"("IN 19:0"="DIO.A_19:0.DIR") -> ("OUT 1:0"=w1179:fxp<+,2,2>, "OUT 3:2"=w1147:fxp<+,2,2>, "OUT 7:4"=w1140:fxp<+,4,4>, "OUT 9:8"=w1098:fxp<+,2,2>, "OUT 11:10"=w1074:fxp<+,2,2>, "OUT 13:12"=w997:fxp<+,2,2>, "OUT 19:18"=w967:fxp<+,2,2>, "OUT 17:16"=w970:fxp<+,2,2>, "OUT 15:14"=w995:fxp<+,2,2>)  [unwired: 6 in]
    n484 = call "Split Function Select.vi"("SYS.SELECT"="SYS.SELECTA") -> ("Selector 1:0"=w1176:fxp<+,4,4>, "Selector 3:2"=w1148:fxp<+,4,4>, "Selector 7:4"=w1139:fxp<+,8,8>, "Selector 9:8"=w1097:fxp<+,4,4>, "Selector 11:10"=w1073:fxp<+,4,4>, "Selector 13:12"=w994:fxp<+,4,4>, "Selector 19:18"=w966:fxp<+,4,4>, "Selector 17:16"=w969:fxp<+,4,4>, "Selector 15:14"=w993:fxp<+,4,4>)  [unwired: 6 in]
    n485 = Bundle By Name(cluster=w1100, "PWM.0.CS"="PWM.A_8.CS", "PWM.0.CNFG"="PWM.A_8.CNFG", "PWM.0.CMP"="PWM.A_8.CMP", "PWM.0.MAX"="PWM.A_8.MAX", "PWM.1.CS"="PWM.A_9.CS", "PWM.1.CNFG"="PWM.A_9.CNFG", "PWM.1.CMP"="PWM.A_9.CMP", "PWM.1.MAX"="PWM.A_9.MAX") -> (w1113:T6)
    n486 = Bundle By Name(cluster=w1109, "ENC.CNFG"="ENC.A_4.CNFG") -> (w1114:T5)
    n487 = Bundle By Name(cluster=w1193, "PWM.0.CS"="PWM.A_0.CS", "PWM.0.CNFG"="PWM.A_0.CNFG", "PWM.0.CMP"="PWM.A_0.CMP", "PWM.0.MAX"="PWM.A_0.MAX", "PWM.1.CS"="PWM.A_1.CS", "PWM.1.CNFG"="PWM.A_1.CNFG", "PWM.1.CMP"="PWM.A_1.CMP", "PWM.1.MAX"="PWM.A_1.MAX") -> (w1178:T6)
    n488 = Bundle By Name(cluster=w1184, "ENC.CNFG"="ENC.A_0.CNFG") -> (w1177:T5)
    n489 = Bundle By Name(cluster=w1162, "PWM.0.CS"="PWM.A_2.CS", "PWM.0.CNFG"="PWM.A_2.CNFG", "PWM.0.CMP"="PWM.A_2.CMP", "PWM.0.MAX"="PWM.A_2.MAX", "PWM.1.CS"="PWM.A_3.CS", "PWM.1.CNFG"="PWM.A_3.CNFG", "PWM.1.CMP"="PWM.A_3.CMP", "PWM.1.MAX"="PWM.A_3.MAX") -> (w1166:T6)
    n490 = Bundle By Name(cluster=w955, "PWM.0.CS"="PWM.A_4.CS", "PWM.0.CNFG"="PWM.A_4.CNFG", "PWM.0.CMP"="PWM.A_4.CMP", "PWM.0.MAX"="PWM.A_4.MAX", "PWM.1.CS"="PWM.A_5.CS", "PWM.1.CNFG"="PWM.A_5.CNFG", "PWM.1.CMP"="PWM.A_5.CMP", "PWM.1.MAX"="PWM.A_5.MAX") -> (w944:T6)
    n491 = Bundle By Name(cluster=w955, "PWM.0.CS"="PWM.A_6.CS", "PWM.0.CNFG"="PWM.A_6.CNFG", "PWM.0.CMP"="PWM.A_6.CMP", "PWM.0.MAX"="PWM.A_6.MAX", "PWM.1.CS"="PWM.A_7.CS", "PWM.1.CNFG"="PWM.A_7.CNFG", "PWM.1.CMP"="PWM.A_7.CMP", "PWM.1.MAX"="PWM.A_7.MAX") -> (w943:T6)
    n492 = Bundle By Name(cluster=w954, "ENC.CNFG"="ENC.A_2.CNFG") -> (w942:T5)
    n493 = Bundle By Name(cluster=w954, "ENC.CNFG"="ENC.A_3.CNFG") -> (w941:T5)
    n494 = Bundle By Name(cluster=w1163, "ENC.CNFG"="ENC.A_1.CNFG") -> (w1167:T5)
    n495 = Bundle By Name(cluster=w1125, "SPI.CNT"="SPI.A.CNT", "SPI.CNFG"="SPI.A.CNFG", "SPI.DATO"="SPI.A.DATO", "SPI.GO"="SPI.A.GO") -> (w957:T8)
    n496 = call "DIO_PWM_Encoder.vi"("DIO.1:0.OUT"=w1099, "DIO.1:0.DIR"=w1098, "PWM.GROUP IN"=w1113, "Encoder.GROUP IN"=w1114, "DIO0/PWM0/ENC.A Refnum"=refnum<k21> "ConnectorA/DIO8" ("FPGA I/O"), "DIO.1:0.Selector"=w1097, "DIO1/PWM1/ENC.B Refnum"=refnum<k21> "ConnectorA/DIO9" ("FPGA I/O")) -> ("IN 1:0"=w963:fxp<+,2,2>, "PWM.GROUP OUT"=w1115:T6, "Encoder.GROUP OUT"=w1118:T5)  [unwired: 10 in]
    n497 = call "DIO_PWM_Encoder.vi"("DIO.1:0.OUT"=w1182, "DIO.1:0.DIR"=w1179, "PWM.GROUP IN"=w1178, "Encoder.GROUP IN"=w1177, "DIO0/PWM0/ENC.A Refnum"=refnum<k21> "ConnectorA/DIO0" ("FPGA I/O"), "DIO.1:0.Selector"=w1176, "DIO1/PWM1/ENC.B Refnum"=refnum<k21> "ConnectorA/DIO1" ("FPGA I/O")) -> ("IN 1:0"=w910:fxp<+,2,2>, "PWM.GROUP OUT"=w1175:T6, "Encoder.GROUP OUT"=w1172:T5)  [unwired: 10 in]
    n498 = call "DIO_PWM_Encoder.vi"("DIO.1:0.OUT"=w1146, "DIO.1:0.DIR"=w1147, "PWM.GROUP IN"=w1166, "Encoder.GROUP IN"=w1167, "DIO0/PWM0/ENC.A Refnum"=refnum<k21> "ConnectorA/DIO2" ("FPGA I/O"), "DIO.1:0.Selector"=w1148, "DIO1/PWM1/ENC.B Refnum"=refnum<k21> "ConnectorA/DIO3" ("FPGA I/O")) -> ("IN 1:0"=w909:fxp<+,2,2>, "PWM.GROUP OUT"=w1168:T6, "Encoder.GROUP OUT"=w1169:T5)  [unwired: 10 in]
    n499 = call "DIO_PWM_Encoder_SPI.vi"("DIO.3:0.OUT"=w1141, "DIO.3:0.DIR"=w1140, "PWM.1:0.GROUP IN"=w944, "PWM.3:2.GROUP IN"=w943, "Encoder.0.GROUP IN"=w942, "Encoder.1.GROUP IN"=w941, "DIO0/PWM0/ENC0.A Refnum"=refnum<k21> "ConnectorA/DIO4" ("FPGA I/O"), "DIO.3:0.Selector"=w1139, "DIO1/PWM1/ENC0.B/SPI.CLK Refnum"=refnum<k21> "ConnectorA/DIO5" ("FPGA I/O"), "SPI.GROUP IN"=w957, "DIO2/PWM2/ENC1.A/SPI.MISO Refnum"=refnum<k21> "ConnectorA/DIO6" ("FPGA I/O"), "DIO3/PWM3/ENC1.B/SPI.MOSI Refnum"=refnum<k21> "ConnectorA/DIO7" ("FPGA I/O")) -> ("SPI.GROUP OUT"=w956:T8, "IN 3:0"=w964:fxp<+,4,4>, "PWM.1:0.GROUP OUT"=w940:T6, "PWM.3:2.GROUP OUT"=w939:T6, "Encoder.0.GROUP OUT"=w938:T5, "Encoder.1.GROUP OUT"=w937:T5)  [unwired: 2 in]
    n500 = Unbundle By Name(w1115) -> ("PWM.0.CNTR"=→"PWM.A_8.CNTR":u16, "PWM.1.CNTR"=→"PWM.A_9.CNTR":u16)
    n501 = Unbundle By Name(w1118) -> ("ENC.CNTR"=→"ENC.A_4.CNTR":u32, "ENC.STAT"=→"ENC.A_4.STAT":u8)
    n502 = Unbundle By Name(w1175) -> ("PWM.0.CNTR"=→"PWM.A_0.CNTR":u16, "PWM.1.CNTR"=→"PWM.A_1.CNTR":u16)
    n503 = Unbundle By Name(w1172) -> ("ENC.CNTR"=→"ENC.A_0.CNTR":u32, "ENC.STAT"=→"ENC.A_0.STAT":u8)
    n504 = Unbundle By Name(w1168) -> ("PWM.0.CNTR"=→"PWM.A_2.CNTR":u16, "PWM.1.CNTR"=→"PWM.A_3.CNTR":u16)
    n505 = Unbundle By Name(w1169) -> ("ENC.CNTR"=→"ENC.A_1.CNTR":u32, "ENC.STAT"=→"ENC.A_1.STAT":u8)
    n506 = Unbundle By Name(w940) -> ("PWM.0.CNTR"=→"PWM.A_4.CNTR":u16, "PWM.1.CNTR"=→"PWM.A_5.CNTR":u16)
    n507 = Unbundle By Name(w939) -> ("PWM.0.CNTR"=→"PWM.A_6.CNTR":u16, "PWM.1.CNTR"=→"PWM.A_7.CNTR":u16)
    n508 = Unbundle By Name(w938) -> ("ENC.CNTR"=→"ENC.A_2.CNTR":u32, "ENC.STAT"=→"ENC.A_2.STAT":u8)
    n509 = Unbundle By Name(w937) -> ("ENC.CNTR"=→"ENC.A_3.CNTR":u32, "ENC.STAT"=→"ENC.A_3.STAT":u8)
    n510 = Unbundle By Name(w956) -> ("SPI.DATI"=→"SPI.A.DATI":u16, "SPI.STAT"=w929:u8)
    "SPI.A.STAT" <- w929
    n511 = Number To Boolean Array(number=w910) -> (Boolean array=w911:bool[])
    n512 = Number To Boolean Array(number=w909) -> (Boolean array=w908:bool[])
    n513 = Number To Boolean Array(number="IRQ.DIO_A_7:0.ENA") -> (Boolean array=w907:bool[])
    n514 = Number To Boolean Array(number="IRQ.DIO_A_7:0.RISE") -> (Boolean array=w906:bool[])
    n515 = Number To Boolean Array(number="IRQ.DIO_A_7:0.FALL") -> (Boolean array=w905:bool[])
    n516 = Index Array(array=w911) -> (element #1=w884:bool, element #2=w883:bool)  [unwired: 2 in]
    n517 = Index Array(array=w908) -> (element #1=w882:bool, element #2=w881:bool)  [unwired: 2 in]
    n518 = Index Array(array=w907) -> (element #1=w901:bool, element #2=w898:bool, element #3=w897:bool, element #4=w896:bool)  [unwired: 4 in]
    n519 = Index Array(array=w906) -> (element #1=w900:bool, element #2=w895:bool, element #3=w894:bool, element #4=w893:bool)  [unwired: 4 in]
    n520 = Index Array(array=w905) -> (element #1=w899:bool, element #2=w892:bool, element #3=w891:bool, element #4=w890:bool)  [unwired: 4 in]
    n521 = Bundle By Name(cluster=w972, "PWM.0.CS"="PWM.A_18.CS", "PWM.0.CNFG"="PWM.A_18.CNFG", "PWM.0.CMP"="PWM.A_18.CMP", "PWM.0.MAX"="PWM.A_18.MAX", "PWM.1.CS"="PWM.A_19.CS", "PWM.1.CNFG"="PWM.A_19.CNFG", "PWM.1.CMP"="PWM.A_19.CMP", "PWM.1.MAX"="PWM.A_19.MAX") -> (w985:T6)
    n522 = Bundle By Name(cluster=w981, "ENC.CNFG"="ENC.A_9.CNFG") -> (w986:T5)
    n523 = Bundle By Name(cluster=w1019, "PWM.0.CS"="PWM.A_16.CS", "PWM.0.CNFG"="PWM.A_16.CNFG", "PWM.0.CMP"="PWM.A_16.CMP", "PWM.0.MAX"="PWM.A_16.MAX", "PWM.1.CS"="PWM.A_17.CS", "PWM.1.CNFG"="PWM.A_17.CNFG", "PWM.1.CMP"="PWM.A_17.CMP", "PWM.1.MAX"="PWM.A_17.MAX") -> (w1006:T6)
    n524 = Bundle By Name(cluster=w1076, "PWM.0.CS"="PWM.A_10.CS", "PWM.0.CNFG"="PWM.A_10.CNFG", "PWM.0.CMP"="PWM.A_10.CMP", "PWM.0.MAX"="PWM.A_10.MAX", "PWM.1.CS"="PWM.A_11.CS", "PWM.1.CNFG"="PWM.A_11.CNFG", "PWM.1.CMP"="PWM.A_11.CMP", "PWM.1.MAX"="PWM.A_11.MAX") -> (w1089:T6)
    n525 = Bundle By Name(cluster=w1072, "PWM.0.CS"="PWM.A_12.CS", "PWM.0.CNFG"="PWM.A_12.CNFG", "PWM.0.CMP"="PWM.A_12.CMP", "PWM.0.MAX"="PWM.A_12.MAX", "PWM.1.CS"="PWM.A_13.CS", "PWM.1.CNFG"="PWM.A_13.CNFG", "PWM.1.CMP"="PWM.A_13.CMP", "PWM.1.MAX"="PWM.A_13.MAX") -> (w1059:T6)
    n526 = Bundle By Name(cluster=w1010, "ENC.CNFG"="ENC.A_8.CNFG") -> (w1005:T5)
    n527 = Bundle By Name(cluster=w1085, "ENC.CNFG"="ENC.A_5.CNFG") -> (w1090:T5)
    n528 = Bundle By Name(cluster=w1032, "PWM.0.CS"="PWM.A_14.CS", "PWM.0.CNFG"="PWM.A_14.CNFG", "PWM.0.CMP"="PWM.A_14.CMP", "PWM.0.MAX"="PWM.A_14.MAX", "PWM.1.CS"="PWM.A_15.CS", "PWM.1.CNFG"="PWM.A_15.CNFG", "PWM.1.CMP"="PWM.A_15.CMP", "PWM.1.MAX"="PWM.A_15.MAX") -> (w1044:T6)
    n529 = Bundle By Name(cluster=w1063, "ENC.CNFG"="ENC.A_6.CNFG") -> (w1058:T5)
    n530 = Bundle By Name(cluster=w1041, "ENC.CNFG"="ENC.A_7.CNFG") -> (w1045:T5)
    n531 = Bundle By Name(cluster=w1030, "I2C.GO"="I2C.A.GO", "I2C.CNFG"="I2C.A.CNFG", "I2C.DATO"="I2C.A.DATO", "I2C.ADDR"="I2C.A.ADDR", "I2C.CNTR"="I2C.A.CNTR", "I2C.CNTL"="I2C.A.CNTL") -> (w1023:T7)
    n532 = call "Check DI IRQ.vi"("Debounce Ticks"=w885, "Count"="IRQ.DIO_A_0.CNT", "On Falling Edge?"=w899, "On Rising Edge?"=w900, "Enable Interrupt?"=w901, "Digital In"=w884) -> ("Trigger?"=w880:bool)  [unwired: 5 in]
    n533 = call "Check DI IRQ.vi"("Debounce Ticks"=w885, "Count"="IRQ.DIO_A_1.CNT", "On Falling Edge?"=w892, "On Rising Edge?"=w895, "Enable Interrupt?"=w898, "Digital In"=w883) -> ("Trigger?"=w879:bool)  [unwired: 5 in]
    n534 = call "Check DI IRQ.vi"("Debounce Ticks"=w885, "Count"="IRQ.DIO_A_2.CNT", "On Falling Edge?"=w891, "On Rising Edge?"=w894, "Enable Interrupt?"=w897, "Digital In"=w882) -> ("Trigger?"=w878:bool)  [unwired: 5 in]
    n535 = feedback #30(w920) -> (w915:u8)
    n536 = Greater?(x=u8 5, y=w915) -> (0:w923:bool)
    n537 = Increment(x=w915) -> (x+1=w922:u8)
    n538 = call "Check DI IRQ.vi"("Debounce Ticks"=w885, "Count"="IRQ.DIO_A_3.CNT", "On Falling Edge?"=w890, "On Rising Edge?"=w893, "Enable Interrupt?"=w896, "Digital In"=w881) -> ("Trigger?"=w877:bool)  [unwired: 5 in]
    n539 = call "DIO_PWM_Encoder.vi"("DIO.1:0.OUT"=w968, "DIO.1:0.DIR"=w967, "PWM.GROUP IN"=w985, "Encoder.GROUP IN"=w986, "DIO0/PWM0/ENC.A Refnum"=refnum<k21> "ConnectorA/DIO18" ("FPGA I/O"), "DIO.1:0.Selector"=w966, "DIO1/PWM1/ENC.B Refnum"=refnum<k21> "ConnectorA/DIO19" ("FPGA I/O")) -> ("IN 1:0"=w958:fxp<+,2,2>, "PWM.GROUP OUT"=w987:T6, "Encoder.GROUP OUT"=w990:T5)  [unwired: 10 in]
    n540 = call "DIO_PWM_Encoder.vi"("DIO.1:0.OUT"=w971, "DIO.1:0.DIR"=w970, "PWM.GROUP IN"=w1006, "Encoder.GROUP IN"=w1005, "DIO0/PWM0/ENC.A Refnum"=refnum<k21> "ConnectorA/DIO16" ("FPGA I/O"), "DIO.1:0.Selector"=w969, "DIO1/PWM1/ENC.B Refnum"=refnum<k21> "ConnectorA/DIO17" ("FPGA I/O")) -> ("IN 1:0"=w959:fxp<+,2,2>, "PWM.GROUP OUT"=w1004:T6, "Encoder.GROUP OUT"=w1001:T5)  [unwired: 10 in]
    n541 = call "DIO_PWM_Encoder.vi"("DIO.1:0.OUT"=w1075, "DIO.1:0.DIR"=w1074, "PWM.GROUP IN"=w1089, "Encoder.GROUP IN"=w1090, "DIO0/PWM0/ENC.A Refnum"=refnum<k21> "ConnectorA/DIO10" ("FPGA I/O"), "DIO.1:0.Selector"=w1073, "DIO1/PWM1/ENC.B Refnum"=refnum<k21> "ConnectorA/DIO11" ("FPGA I/O")) -> ("IN 1:0"=w962:fxp<+,2,2>, "PWM.GROUP OUT"=w1091:T6, "Encoder.GROUP OUT"=w1094:T5)  [unwired: 10 in]
    n542 = call "DIO_PWM_Encoder.vi"("DIO.1:0.OUT"=w998, "DIO.1:0.DIR"=w997, "PWM.GROUP IN"=w1059, "Encoder.GROUP IN"=w1058, "DIO0/PWM0/ENC.A Refnum"=refnum<k21> "ConnectorA/DIO12" ("FPGA I/O"), "DIO.1:0.Selector"=w994, "DIO1/PWM1/ENC.B Refnum"=refnum<k21> "ConnectorA/DIO13" ("FPGA I/O")) -> ("IN 1:0"=w961:fxp<+,2,2>, "PWM.GROUP OUT"=w1057:T6, "Encoder.GROUP OUT"=w1054:T5)  [unwired: 10 in]
    n543 = call "DIO_PWM_Encoder_I2C.vi"("DIO.1:0.OUT"=w996, "DIO.1:0.DIR"=w995, "PWM.GROUP IN"=w1044, "Encoder.GROUP IN"=w1045, "I2C.GROUP IN"=w1023, "DIO0/PWM0/ENC.A/I2C.SCL Refnum"=refnum<k21> "ConnectorA/DIO14" ("FPGA I/O"), "DIO.1:0.Selector"=w993, "DIO1/PWM1/ENC.B/I2C.SDA Refnum"=refnum<k21> "ConnectorA/DIO15" ("FPGA I/O")) -> ("IN 1:0"=w960:fxp<+,2,2>, "PWM.GROUP OUT"=w1046:T6, "Encoder.GROUP OUT"=w1049:T5, "I2C.GROUP OUT"=w1022:T7)  [unwired: 8 in]
    n544 = Select(t=w922, s=w923, f=w920) -> (s? t:f=w921:u8)
    n545 = feedback-in #30(w921) -> ()
    n546 = Unbundle By Name(w987) -> ("PWM.0.CNTR"=→"PWM.A_18.CNTR":u16, "PWM.1.CNTR"=→"PWM.A_19.CNTR":u16)
    n547 = Unbundle By Name(w990) -> ("ENC.CNTR"=→"ENC.A_9.CNTR":u32, "ENC.STAT"=→"ENC.A_9.STAT":u8)
    n548 = Unbundle By Name(w1004) -> ("PWM.0.CNTR"=→"PWM.A_16.CNTR":u16, "PWM.1.CNTR"=→"PWM.A_17.CNTR":u16)
    n549 = Unbundle By Name(w1091) -> ("PWM.0.CNTR"=→"PWM.A_10.CNTR":u16, "PWM.1.CNTR"=→"PWM.A_11.CNTR":u16)
    n550 = Unbundle By Name(w1001) -> ("ENC.CNTR"=→"ENC.A_8.CNTR":u32, "ENC.STAT"=→"ENC.A_8.STAT":u8)
    n551 = Unbundle By Name(w1094) -> ("ENC.CNTR"=→"ENC.A_5.CNTR":u32, "ENC.STAT"=→"ENC.A_5.STAT":u8)
    n552 = Unbundle By Name(w1057) -> ("PWM.0.CNTR"=→"PWM.A_12.CNTR":u16, "PWM.1.CNTR"=→"PWM.A_13.CNTR":u16)
    n553 = Unbundle By Name(w1054) -> ("ENC.CNTR"=→"ENC.A_6.CNTR":u32, "ENC.STAT"=→"ENC.A_6.STAT":u8)
    n554 = Unbundle By Name(w1046) -> ("PWM.0.CNTR"=→"PWM.A_14.CNTR":u16, "PWM.1.CNTR"=→"PWM.A_15.CNTR":u16)
    n555 = Unbundle By Name(w1049) -> ("ENC.CNTR"=→"ENC.A_7.CNTR":u32, "ENC.STAT"=→"ENC.A_7.STAT":u8)
    n556 = case shown="0, 默认" w915 {
      tunnel: ["IRQ.DIO_A_0.NO" "IRQ.DIO_A_1.NO" "IRQ.DIO_A_2.NO" "IRQ.DIO_A_3.NO" w1212 w1213] -> w914
      frame 0, Default {
        # "DI0 IRQ"
      }
      frame 1 {
        # "DI1 IRQ"
      }
      frame 2 {
        # "DI2 IRQ"
      }
      frame 3 {
        # "DI3 IRQ"
      }
      frame 4 {
        # "SPI IRQ"
        n557 = global read "ELVIS III Global.vi" "SPI.A.IRQ_NO"() -> (w1212:u8)
      }
      frame 5 {
        # "DO Block IRQ"
        n558 = global read "ELVIS III Global.vi" "DO.A.DMA_IRQ_NO"() -> (w1213:u8)
      }
    }
    n559 = Unbundle By Name(w1022) -> ("I2C.DATI"=→"I2C.A.DATI":u8, "I2C.STAT"=→"I2C.A.STAT":u8)
    n560 = Number To Boolean Array(number=w929) -> (Boolean array=w931:bool[])
    n561 = Index Array(array=w931) -> (element=w930:bool)  [unwired: 1 in]
    n562 = call "Falling Edge Trigger.vi"("Signal"=w930) -> ("Trigger?"=w928:bool)
    n563 = call "Rising Edge Trigger.vi"("Signal"=w1197) -> ("Trigger?"=w927:bool)
    n564 = Build Array(w880, w879, w878, w877, w928, w927) -> (w925:bool[])
    n565 = call "Join Bank DIO.vi"("IN 7:4"=w964, "IN 3:2"=w909, "IN 1:0"=w910, "IN 9:8"=w963, "IN 11:10"=w962, "IN 13:12"=w961, "IN 15:14"=w960, "IN 17:16"=w959, "IN 19:18"=w958) -> ("OUT 19:0"=w965:fxp<+,20,20>)  [unwired: 6 in]
    n566 = xnode "FPGA I/O Node"() -> ("错误输出"=w913:errorcluster)  [unwired: 2 in, 2 out]
    n567 = feedback #31(bool[] [FALSE, FALSE, FALSE, FALSE, FALSE, FALSE]) -> (w1198:bool[])
    n568 = Or(x=w925, y=w1198) -> (x .or. y?=w918:bool[])
    n569 = Index Array(array=w918, index=w915) -> (element=w919:bool)
    n570 = case shown="真" w919 {
      selector: w919 -> [w1214 _]
      tunnel: [w1214 w1216] -> w917
      tunnel: w914 -> [_ w1215]
      frame False {
      }
      frame True {
        n571 = xnode ("FIFO Write")("元素"=w1215, "超时"=0 ("Timeout")) -> ("超时？"=w1216:bool)  [unwired: 1 in, 1 out]
      }
    }
    n572 = call "DIO Read Bank.vi"("DI.DMA_ENA"="DI.A.DMA_ENA", "DI.DMA_CNTR"="DI.A.DMA_CNTR", "DATA IN"=w965, "DMA FIFO IN"=refnum<k21> "DI.A.DMA" ("FIFO")) -> ("DI.DMA_IDL"=→"DI.A.DMA_IDL":bool, "DIO.A_0:15.IN"=→"DIO.A_19:0.IN":fxp<+,20,20>)  [unwired: 6 in]
    n573 = Unbundle By Name(w913) -> ("status"=→"UART.A.STAT":bool)
    n574 = Replace Array Subset(array=w918, new element=w917, index=w915) -> (w916:bool[])
    n575 = feedback-in #31(w916) -> ()
  }
  n576 = node-c288(w21) -> ()
  n577 = node-c288() -> (w20:T2)  [unwired: 1 in]
  n578 = timed-loop {
    timing: w20 -> [_]
    timing-out: [_] -> w19
    stop <- _ stop-if-true
    w1234 = u8 0
    w1292 = T5 {"ENC.CNFG"=0, "ENC.CNTR"=0, "ENC.STAT"=0}  # Encoder.GROUP
    w1283 = T6 {"PWM.0.CS"=0, "PWM.0.CNFG"=0, "PWM.0.CMP"=0, "PWM.0.MAX"=0, "PWM.0.CNTR"=0, "PWM.1.CS"=0, "PWM.1.CNFG"=0, "PWM.1.CMP"=0, "PWM.1.MAX"=0, "PWM.1.CNTR"=0}  # PWM.GROUP
    w1321 = T5 {"ENC.CNFG"=0, "ENC.CNTR"=0, "ENC.STAT"=0}  # Encoder.GROUP
    w1330 = T6 {"PWM.0.CS"=0, "PWM.0.CNFG"=0, "PWM.0.CMP"=0, "PWM.0.MAX"=0, "PWM.0.CNTR"=0, "PWM.1.CS"=0, "PWM.1.CNFG"=0, "PWM.1.CMP"=0, "PWM.1.MAX"=0, "PWM.1.CNTR"=0}  # PWM.GROUP
    w1341 = T7 {"I2C.GO"=FALSE, "I2C.CNFG"=1, "I2C.DATO"=0, "I2C.DATI"=0, "I2C.ADDR"=0, "I2C.CNTR"=213, "I2C.CNTL"=0, "I2C.STAT"=0}  # I2C.GROUP
    w1352 = T5 {"ENC.CNFG"=0, "ENC.CNTR"=0, "ENC.STAT"=0}  # Encoder.GROUP
    w1343 = T6 {"PWM.0.CS"=0, "PWM.0.CNFG"=0, "PWM.0.CMP"=0, "PWM.0.MAX"=0, "PWM.0.CNTR"=0, "PWM.1.CS"=0, "PWM.1.CNFG"=0, "PWM.1.CMP"=0, "PWM.1.MAX"=0, "PWM.1.CNTR"=0}  # PWM.GROUP
    w1374 = T5 {"ENC.CNFG"=0, "ENC.CNTR"=0, "ENC.STAT"=0}  # Encoder.GROUP
    w1383 = T6 {"PWM.0.CS"=0, "PWM.0.CNFG"=0, "PWM.0.CMP"=0, "PWM.0.MAX"=0, "PWM.0.CNTR"=0, "PWM.1.CS"=0, "PWM.1.CNFG"=0, "PWM.1.CMP"=0, "PWM.1.MAX"=0, "PWM.1.CNTR"=0}  # PWM.GROUP
    w1396 = T5 {"ENC.CNFG"=0, "ENC.CNTR"=0, "ENC.STAT"=0}  # Encoder.GROUP
    w1387 = T6 {"PWM.0.CS"=0, "PWM.0.CNFG"=0, "PWM.0.CMP"=0, "PWM.0.MAX"=0, "PWM.0.CNTR"=0, "PWM.1.CS"=0, "PWM.1.CNFG"=0, "PWM.1.CMP"=0, "PWM.1.MAX"=0, "PWM.1.CNTR"=0}  # PWM.GROUP
    w1420 = T5 {"ENC.CNFG"=0, "ENC.CNTR"=0, "ENC.STAT"=0}  # Encoder.GROUP
    w1411 = T6 {"PWM.0.CS"=0, "PWM.0.CNFG"=0, "PWM.0.CMP"=0, "PWM.0.MAX"=0, "PWM.0.CNTR"=0, "PWM.1.CS"=0, "PWM.1.CNFG"=0, "PWM.1.CMP"=0, "PWM.1.MAX"=0, "PWM.1.CNTR"=0}  # PWM.GROUP
    w1436 = T8 {"SPI.STAT"=0, "SPI.GO"=FALSE, "SPI.CNT"=19, "SPI.CNFG"=112, "SPI.DATI"=0, "SPI.DATO"=0}  # SPI.GROUP
    w1257 = T5 {"ENC.CNFG"=0, "ENC.CNTR"=0, "ENC.STAT"=0}  # Encoder.GROUP
    w1266 = T6 {"PWM.0.CS"=0, "PWM.0.CNFG"=0, "PWM.0.CMP"=0, "PWM.0.MAX"=0, "PWM.0.CNTR"=0, "PWM.1.CS"=0, "PWM.1.CNFG"=0, "PWM.1.CMP"=0, "PWM.1.MAX"=0, "PWM.1.CNTR"=0}  # PWM.GROUP
    w1475 = T5 {"ENC.CNFG"=0, "ENC.CNTR"=0, "ENC.STAT"=0}  # Encoder.GROUP
    w1474 = T6 {"PWM.0.CS"=0, "PWM.0.CNFG"=0, "PWM.0.CMP"=0, "PWM.0.MAX"=0, "PWM.0.CNTR"=0, "PWM.1.CS"=0, "PWM.1.CNFG"=0, "PWM.1.CMP"=0, "PWM.1.MAX"=0, "PWM.1.CNTR"=0}  # PWM.GROUP
    w1496 = T5 {"ENC.CNFG"=0, "ENC.CNTR"=0, "ENC.STAT"=0}  # Encoder.GROUP
    w1505 = T6 {"PWM.0.CS"=0, "PWM.0.CNFG"=0, "PWM.0.CMP"=0, "PWM.0.MAX"=0, "PWM.0.CNTR"=0, "PWM.1.CS"=0, "PWM.1.CNFG"=0, "PWM.1.CMP"=0, "PWM.1.MAX"=0, "PWM.1.CNTR"=0}  # PWM.GROUP
    # "DIO/UART Error Handling"
    # "DIO/PWM/Encoder"
    # "DIO/PWM/Encoder"
    # "DIO/PWM/Encoder/I2C"
    # "DIO/PWM/Encoder"
    # "DIO/PWM/Encoder"
    # ">>B.DIO_19:0.OUT>>"
    # "DIO/PWM/Encoder"
    # "DIO/PWM/Encoder/SPI"
    # "DIO/PWM/Encoder"
    # "DIO/PWM/Encoder"
    # "TODO:\nAdd DIO INT here."
    # "Write DIO"
    # "Read DIO"
    # "DIO Bank B"
    n579 = call "DIO Write Bank.vi"("DIO.19:0.OUT"="DIO.B_19:0.OUT", "DO.DMA_CNTR"="DO.B.DMA_CNTR", "DO.DMA_ENA"="DO.B.DMA_ENA", "DMA FIFO IN"=refnum<k21> "DO.B.DMA" ("DMA FIFO In")) -> ("DO.DMA_IDL"=w1227:bool, "DATA OUT"=w1506:fxp<+,20,20>)  [unwired: 6 in]
    "DO.B.DMA_IDL" <- w1227
    n580 = call "Split Bank DIO.vi"("IN 19:0"=w1506) -> ("OUT 1:0"=w1494:fxp<+,2,2>, "OUT 3:2"=w1458:fxp<+,2,2>, "OUT 7:4"=w1453:fxp<+,4,4>, "OUT 9:8"=w1410:fxp<+,2,2>, "OUT 11:10"=w1386:fxp<+,2,2>, "OUT 13:12"=w1309:fxp<+,2,2>, "OUT 19:18"=w1279:fxp<+,2,2>, "OUT 17:16"=w1282:fxp<+,2,2>, "OUT 15:14"=w1307:fxp<+,2,2>)  [unwired: 6 in]
    n581 = call "Split Bank DIO.vi"("IN 19:0"="DIO.B_19:0.DIR") -> ("OUT 1:0"=w1491:fxp<+,2,2>, "OUT 3:2"=w1459:fxp<+,2,2>, "OUT 7:4"=w1452:fxp<+,4,4>, "OUT 9:8"=w1409:fxp<+,2,2>, "OUT 11:10"=w1385:fxp<+,2,2>, "OUT 13:12"=w1308:fxp<+,2,2>, "OUT 19:18"=w1278:fxp<+,2,2>, "OUT 17:16"=w1281:fxp<+,2,2>, "OUT 15:14"=w1306:fxp<+,2,2>)  [unwired: 6 in]
    n582 = call "Split Function Select.vi"("SYS.SELECT"="SYS.SELECTB") -> ("Selector 1:0"=w1488:fxp<+,4,4>, "Selector 3:2"=w1460:fxp<+,4,4>, "Selector 7:4"=w1451:fxp<+,8,8>, "Selector 9:8"=w1408:fxp<+,4,4>, "Selector 11:10"=w1384:fxp<+,4,4>, "Selector 13:12"=w1305:fxp<+,4,4>, "Selector 19:18"=w1277:fxp<+,4,4>, "Selector 17:16"=w1280:fxp<+,4,4>, "Selector 15:14"=w1304:fxp<+,4,4>)  [unwired: 6 in]
    n583 = Bundle By Name(cluster=w1411, "PWM.0.CS"="PWM.B_8.CS", "PWM.0.CNFG"="PWM.B_8.CNFG", "PWM.0.CMP"="PWM.B_8.CMP", "PWM.0.MAX"="PWM.B_8.MAX", "PWM.1.CS"="PWM.B_9.CS", "PWM.1.CNFG"="PWM.B_9.CNFG", "PWM.1.CMP"="PWM.B_9.CMP", "PWM.1.MAX"="PWM.B_9.MAX") -> (w1424:T6)
    n584 = Bundle By Name(cluster=w1420, "ENC.CNFG"="ENC.B_4.CNFG") -> (w1425:T5)
    n585 = Bundle By Name(cluster=w1505, "PWM.0.CS"="PWM.B_0.CS", "PWM.0.CNFG"="PWM.B_0.CNFG", "PWM.0.CMP"="PWM.B_0.CMP", "PWM.0.MAX"="PWM.B_0.MAX", "PWM.1.CS"="PWM.B_1.CS", "PWM.1.CNFG"="PWM.B_1.CNFG", "PWM.1.CMP"="PWM.B_1.CMP", "PWM.1.MAX"="PWM.B_1.MAX") -> (w1490:T6)
    n586 = Bundle By Name(cluster=w1496, "ENC.CNFG"="ENC.B_0.CNFG") -> (w1489:T5)
    n587 = Bundle By Name(cluster=w1474, "PWM.0.CS"="PWM.B_2.CS", "PWM.0.CNFG"="PWM.B_2.CNFG", "PWM.0.CMP"="PWM.B_2.CMP", "PWM.0.MAX"="PWM.B_2.MAX", "PWM.1.CS"="PWM.B_3.CS", "PWM.1.CNFG"="PWM.B_3.CNFG", "PWM.1.CMP"="PWM.B_3.CMP", "PWM.1.MAX"="PWM.B_3.MAX") -> (w1478:T6)
    n588 = Bundle By Name(cluster=w1266, "PWM.0.CS"="PWM.B_4.CS", "PWM.0.CNFG"="PWM.B_4.CNFG", "PWM.0.CMP"="PWM.B_4.CMP", "PWM.0.MAX"="PWM.B_4.MAX", "PWM.1.CS"="PWM.B_5.CS", "PWM.1.CNFG"="PWM.B_5.CNFG", "PWM.1.CMP"="PWM.B_5.CMP", "PWM.1.MAX"="PWM.B_5.MAX") -> (w1222:T6)
    n589 = Bundle By Name(cluster=w1266, "PWM.0.CS"="PWM.B_6.CS", "PWM.0.CNFG"="PWM.B_6.CNFG", "PWM.0.CMP"="PWM.B_6.CMP", "PWM.0.MAX"="PWM.B_6.MAX", "PWM.1.CS"="PWM.B_7.CS", "PWM.1.CNFG"="PWM.B_7.CNFG", "PWM.1.CMP"="PWM.B_7.CMP", "PWM.1.MAX"="PWM.B_7.MAX") -> (w1221:T6)
    n590 = Bundle By Name(cluster=w1257, "ENC.CNFG"="ENC.B_2.CNFG") -> (w1437:T5)
    n591 = Bundle By Name(cluster=w1257, "ENC.CNFG"="ENC.B_3.CNFG") -> (w1220:T5)
    n592 = Bundle By Name(cluster=w1475, "ENC.CNFG"="ENC.B_1.CNFG") -> (w1479:T5)
    n593 = Bundle By Name(cluster=w1436, "SPI.CNT"="SPI.B.CNT", "SPI.CNFG"="SPI.B.CNFG", "SPI.DATO"="SPI.B.DATO", "SPI.GO"="SPI.B.GO") -> (w1250:T8)
    n594 = call "DIO_PWM_Encoder.vi"("DIO.1:0.OUT"=w1410, "DIO.1:0.DIR"=w1409, "PWM.GROUP IN"=w1424, "Encoder.GROUP IN"=w1425, "DIO0/PWM0/ENC.A Refnum"=refnum<k21> "ConnectorB/DIO8" ("FPGA I/O"), "DIO.1:0.Selector"=w1408, "DIO1/PWM1/ENC.B Refnum"=refnum<k21> "ConnectorB/DIO9" ("FPGA I/O")) -> ("IN 1:0"=w1272:fxp<+,2,2>, "PWM.GROUP OUT"=w1426:T6, "Encoder.GROUP OUT"=w1429:T5)  [unwired: 10 in]
    n595 = call "DIO_PWM_Encoder.vi"("DIO.1:0.OUT"=w1494, "DIO.1:0.DIR"=w1491, "PWM.GROUP IN"=w1490, "Encoder.GROUP IN"=w1489, "DIO0/PWM0/ENC.A Refnum"=refnum<k21> "ConnectorB/DIO0" ("FPGA I/O"), "DIO.1:0.Selector"=w1488, "DIO1/PWM1/ENC.B Refnum"=refnum<k21> "ConnectorB/DIO1" ("FPGA I/O")) -> ("IN 1:0"=w1275:fxp<+,2,2>, "PWM.GROUP OUT"=w1487:T6, "Encoder.GROUP OUT"=w1484:T5)  [unwired: 10 in]
    n596 = call "DIO_PWM_Encoder.vi"("DIO.1:0.OUT"=w1458, "DIO.1:0.DIR"=w1459, "PWM.GROUP IN"=w1478, "Encoder.GROUP IN"=w1479, "DIO0/PWM0/ENC.A Refnum"=refnum<k21> "ConnectorB/DIO2" ("FPGA I/O"), "DIO.1:0.Selector"=w1460, "DIO1/PWM1/ENC.B Refnum"=refnum<k21> "ConnectorB/DIO3" ("FPGA I/O")) -> ("IN 1:0"=w1274:fxp<+,2,2>, "PWM.GROUP OUT"=w1480:T6, "Encoder.GROUP OUT"=w1481:T5)  [unwired: 10 in]
    n597 = call "DIO_PWM_Encoder_SPI.vi"("DIO.3:0.OUT"=w1453, "DIO.3:0.DIR"=w1452, "PWM.1:0.GROUP IN"=w1222, "PWM.3:2.GROUP IN"=w1221, "Encoder.0.GROUP IN"=w1437, "Encoder.1.GROUP IN"=w1220, "DIO0/PWM0/ENC0.A Refnum"=refnum<k21> "ConnectorB/DIO4" ("FPGA I/O"), "DIO.3:0.Selector"=w1451, "DIO1/PWM1/ENC0.B/SPI.CLK Refnum"=refnum<k21> "ConnectorB/DIO5" ("FPGA I/O"), "SPI.GROUP IN"=w1250, "DIO2/PWM2/ENC1.A/SPI.MISO Refnum"=refnum<k21> "ConnectorB/DIO6" ("FPGA I/O"), "DIO3/PWM3/ENC1.B/SPI.MOSI Refnum"=refnum<k21> "ConnectorB/DIO7" ("FPGA I/O")) -> ("SPI.GROUP OUT"=w1251:T8, "IN 3:0"=w1273:fxp<+,4,4>, "PWM.1:0.GROUP OUT"=w1255:T6, "PWM.3:2.GROUP OUT"=w1254:T6, "Encoder.0.GROUP OUT"=w1253:T5, "Encoder.1.GROUP OUT"=w1252:T5)  [unwired: 2 in]
    n598 = Unbundle By Name(w1426) -> ("PWM.0.CNTR"=→"PWM.B_8.CNTR":u16, "PWM.1.CNTR"=→"PWM.B_9.CNTR":u16)
    n599 = Unbundle By Name(w1429) -> ("ENC.CNTR"=→"ENC.B_4.CNTR":u32, "ENC.STAT"=→"ENC.B_4.STAT":u8)
    n600 = Unbundle By Name(w1487) -> ("PWM.0.CNTR"=→"PWM.B_0.CNTR":u16, "PWM.1.CNTR"=→"PWM.B_1.CNTR":u16)
    n601 = Unbundle By Name(w1484) -> ("ENC.CNTR"=→"ENC.B_0.CNTR":u32, "ENC.STAT"=→"ENC.B_0.STAT":u8)
    n602 = Unbundle By Name(w1480) -> ("PWM.0.CNTR"=→"PWM.B_2.CNTR":u16, "PWM.1.CNTR"=→"PWM.B_3.CNTR":u16)
    n603 = Unbundle By Name(w1481) -> ("ENC.CNTR"=→"ENC.B_1.CNTR":u32, "ENC.STAT"=→"ENC.B_1.STAT":u8)
    n604 = Unbundle By Name(w1255) -> ("PWM.0.CNTR"=→"PWM.B_4.CNTR":u16, "PWM.1.CNTR"=→"PWM.B_5.CNTR":u16)
    n605 = Unbundle By Name(w1254) -> ("PWM.0.CNTR"=→"PWM.B_6.CNTR":u16, "PWM.1.CNTR"=→"PWM.B_7.CNTR":u16)
    n606 = Unbundle By Name(w1253) -> ("ENC.CNTR"=→"ENC.B_2.CNTR":u32, "ENC.STAT"=→"ENC.B_2.STAT":u8)
    n607 = Unbundle By Name(w1252) -> ("ENC.CNTR"=→"ENC.B_3.CNTR":u32, "ENC.STAT"=→"ENC.B_3.STAT":u8)
    n608 = Unbundle By Name(w1251) -> ("SPI.DATI"=→"SPI.B.DATI":u16, "SPI.STAT"=w1225:u8)
    "SPI.B.STAT" <- w1225
    n609 = feedback #32(w1234) -> (w1229:u8)
    n610 = Greater?(x=u8 1, y=w1229) -> (0:w1237:bool)
    n611 = Increment(x=w1229) -> (x+1=w1236:u8)
    n612 = Number To Boolean Array(number=w1225) -> (Boolean array=w1244:bool[])
    n613 = Select(t=w1236, s=w1237, f=w1234) -> (s? t:f=w1235:u8)
    n614 = feedback-in #32(w1235) -> ()
    n615 = case shown="1" w1229 {
      tunnel: [w1518 w1519] -> w1228
      frame 0, Default {
        # "SPI IRQ"
        n616 = global read "ELVIS III Global.vi" "SPI.B.IRQ_NO"() -> (w1518:u8)
      }
      frame 1 {
        # "DO Block IRQ"
        n617 = global read "ELVIS III Global.vi" "DO.B.DMA_IRQ_NO"() -> (w1519:u8)
      }
    }
    n618 = Index Array(array=w1244) -> (element=w1243:bool)  [unwired: 1 in]
    n619 = call "Falling Edge Trigger.vi"("Signal"=w1243) -> ("Trigger?"=w1242:bool)
    n620 = call "Rising Edge Trigger.vi"("Signal"=w1227) -> ("Trigger?"=w1241:bool)
    n621 = Build Array(w1242, w1241) -> (w1239:bool[])
    n622 = Bundle By Name(cluster=w1283, "PWM.0.CS"="PWM.B_18.CS", "PWM.0.CNFG"="PWM.B_18.CNFG", "PWM.0.CMP"="PWM.B_18.CMP", "PWM.0.MAX"="PWM.B_18.MAX", "PWM.1.CS"="PWM.B_19.CS", "PWM.1.CNFG"="PWM.B_19.CNFG", "PWM.1.CMP"="PWM.B_19.CMP", "PWM.1.MAX"="PWM.B_19.MAX") -> (w1296:T6)
    n623 = Bundle By Name(cluster=w1292, "ENC.CNFG"="ENC.B_9.CNFG") -> (w1297:T5)
    n624 = Bundle By Name(cluster=w1330, "PWM.0.CS"="PWM.B_16.CS", "PWM.0.CNFG"="PWM.B_16.CNFG", "PWM.0.CMP"="PWM.B_16.CMP", "PWM.0.MAX"="PWM.B_16.MAX", "PWM.1.CS"="PWM.B_17.CS", "PWM.1.CNFG"="PWM.B_17.CNFG", "PWM.1.CMP"="PWM.B_17.CMP", "PWM.1.MAX"="PWM.B_17.MAX") -> (w1317:T6)
    n625 = Bundle By Name(cluster=w1387, "PWM.0.CS"="PWM.B_10.CS", "PWM.0.CNFG"="PWM.B_10.CNFG", "PWM.0.CMP"="PWM.B_10.CMP", "PWM.0.MAX"="PWM.B_10.MAX", "PWM.1.CS"="PWM.B_11.CS", "PWM.1.CNFG"="PWM.B_11.CNFG", "PWM.1.CMP"="PWM.B_11.CMP", "PWM.1.MAX"="PWM.B_11.MAX") -> (w1400:T6)
    n626 = Bundle By Name(cluster=w1383, "PWM.0.CS"="PWM.B_12.CS", "PWM.0.CNFG"="PWM.B_12.CNFG", "PWM.0.CMP"="PWM.B_12.CMP", "PWM.0.MAX"="PWM.B_12.MAX", "PWM.1.CS"="PWM.B_13.CS", "PWM.1.CNFG"="PWM.B_13.CNFG", "PWM.1.CMP"="PWM.B_13.CMP", "PWM.1.MAX"="PWM.B_13.MAX") -> (w1370:T6)
    n627 = Bundle By Name(cluster=w1321, "ENC.CNFG"="ENC.B_8.CNFG") -> (w1316:T5)
    n628 = Bundle By Name(cluster=w1396, "ENC.CNFG"="ENC.B_5.CNFG") -> (w1401:T5)
    n629 = Bundle By Name(cluster=w1343, "PWM.0.CS"="PWM.B_14.CS", "PWM.0.CNFG"="PWM.B_14.CNFG", "PWM.0.CMP"="PWM.B_14.CMP", "PWM.0.MAX"="PWM.B_14.MAX", "PWM.1.CS"="PWM.B_15.CS", "PWM.1.CNFG"="PWM.B_15.CNFG", "PWM.1.CMP"="PWM.B_15.CMP", "PWM.1.MAX"="PWM.B_15.MAX") -> (w1355:T6)
    n630 = Bundle By Name(cluster=w1374, "ENC.CNFG"="ENC.B_6.CNFG") -> (w1369:T5)
    n631 = Bundle By Name(cluster=w1352, "ENC.CNFG"="ENC.B_7.CNFG") -> (w1356:T5)
    n632 = Bundle By Name(cluster=w1341, "I2C.GO"="I2C.B.GO", "I2C.CNFG"="I2C.B.CNFG", "I2C.DATO"="I2C.B.DATO", "I2C.ADDR"="I2C.B.ADDR", "I2C.CNTR"="I2C.B.CNTR", "I2C.CNTL"="I2C.B.CNTL") -> (w1334:T7)
    n633 = call "DIO_PWM_Encoder.vi"("DIO.1:0.OUT"=w1279, "DIO.1:0.DIR"=w1278, "PWM.GROUP IN"=w1296, "Encoder.GROUP IN"=w1297, "DIO0/PWM0/ENC.A Refnum"=refnum<k21> "ConnectorB/DIO18" ("FPGA I/O"), "DIO.1:0.Selector"=w1277, "DIO1/PWM1/ENC.B Refnum"=refnum<k21> "ConnectorB/DIO19" ("FPGA I/O")) -> ("IN 1:0"=w1267:fxp<+,2,2>, "PWM.GROUP OUT"=w1298:T6, "Encoder.GROUP OUT"=w1301:T5)  [unwired: 10 in]
    n634 = call "DIO_PWM_Encoder.vi"("DIO.1:0.OUT"=w1282, "DIO.1:0.DIR"=w1281, "PWM.GROUP IN"=w1317, "Encoder.GROUP IN"=w1316, "DIO0/PWM0/ENC.A Refnum"=refnum<k21> "ConnectorB/DIO16" ("FPGA I/O"), "DIO.1:0.Selector"=w1280, "DIO1/PWM1/ENC.B Refnum"=refnum<k21> "ConnectorB/DIO17" ("FPGA I/O")) -> ("IN 1:0"=w1268:fxp<+,2,2>, "PWM.GROUP OUT"=w1315:T6, "Encoder.GROUP OUT"=w1312:T5)  [unwired: 10 in]
    n635 = call "DIO_PWM_Encoder.vi"("DIO.1:0.OUT"=w1386, "DIO.1:0.DIR"=w1385, "PWM.GROUP IN"=w1400, "Encoder.GROUP IN"=w1401, "DIO0/PWM0/ENC.A Refnum"=refnum<k21> "ConnectorB/DIO10" ("FPGA I/O"), "DIO.1:0.Selector"=w1384, "DIO1/PWM1/ENC.B Refnum"=refnum<k21> "ConnectorB/DIO11" ("FPGA I/O")) -> ("IN 1:0"=w1271:fxp<+,2,2>, "PWM.GROUP OUT"=w1402:T6, "Encoder.GROUP OUT"=w1405:T5)  [unwired: 10 in]
    n636 = call "DIO_PWM_Encoder.vi"("DIO.1:0.OUT"=w1309, "DIO.1:0.DIR"=w1308, "PWM.GROUP IN"=w1370, "Encoder.GROUP IN"=w1369, "DIO0/PWM0/ENC.A Refnum"=refnum<k21> "ConnectorB/DIO12" ("FPGA I/O"), "DIO.1:0.Selector"=w1305, "DIO1/PWM1/ENC.B Refnum"=refnum<k21> "ConnectorB/DIO13" ("FPGA I/O")) -> ("IN 1:0"=w1270:fxp<+,2,2>, "PWM.GROUP OUT"=w1368:T6, "Encoder.GROUP OUT"=w1365:T5)  [unwired: 10 in]
    n637 = call "DIO_PWM_Encoder_I2C.vi"("DIO.1:0.OUT"=w1307, "DIO.1:0.DIR"=w1306, "PWM.GROUP IN"=w1355, "Encoder.GROUP IN"=w1356, "I2C.GROUP IN"=w1334, "DIO0/PWM0/ENC.A/I2C.SCL Refnum"=refnum<k21> "ConnectorB/DIO14" ("FPGA I/O"), "DIO.1:0.Selector"=w1304, "DIO1/PWM1/ENC.B/I2C.SDA Refnum"=refnum<k21> "ConnectorB/DIO15" ("FPGA I/O")) -> ("IN 1:0"=w1269:fxp<+,2,2>, "PWM.GROUP OUT"=w1357:T6, "Encoder.GROUP OUT"=w1360:T5, "I2C.GROUP OUT"=w1333:T7)  [unwired: 8 in]
    n638 = Unbundle By Name(w1298) -> ("PWM.0.CNTR"=→"PWM.B_18.CNTR":u16, "PWM.1.CNTR"=→"PWM.B_19.CNTR":u16)
    n639 = Unbundle By Name(w1301) -> ("ENC.CNTR"=→"ENC.B_9.CNTR":u32, "ENC.STAT"=→"ENC.B_9.STAT":u8)
    n640 = Unbundle By Name(w1315) -> ("PWM.0.CNTR"=→"PWM.B_16.CNTR":u16, "PWM.1.CNTR"=→"PWM.B_17.CNTR":u16)
    n641 = Unbundle By Name(w1402) -> ("PWM.0.CNTR"=→"PWM.B_10.CNTR":u16, "PWM.1.CNTR"=→"PWM.B_11.CNTR":u16)
    n642 = Unbundle By Name(w1312) -> ("ENC.CNTR"=→"ENC.B_8.CNTR":u32, "ENC.STAT"=→"ENC.B_8.STAT":u8)
    n643 = Unbundle By Name(w1405) -> ("ENC.CNTR"=→"ENC.B_5.CNTR":u32, "ENC.STAT"=→"ENC.B_5.STAT":u8)
    n644 = Unbundle By Name(w1368) -> ("PWM.0.CNTR"=→"PWM.B_12.CNTR":u16, "PWM.1.CNTR"=→"PWM.B_13.CNTR":u16)
    n645 = Unbundle By Name(w1365) -> ("ENC.CNTR"=→"ENC.B_6.CNTR":u32, "ENC.STAT"=→"ENC.B_6.STAT":u8)
    n646 = Unbundle By Name(w1357) -> ("PWM.0.CNTR"=→"PWM.B_14.CNTR":u16, "PWM.1.CNTR"=→"PWM.B_15.CNTR":u16)
    n647 = Unbundle By Name(w1360) -> ("ENC.CNTR"=→"ENC.B_7.CNTR":u32, "ENC.STAT"=→"ENC.B_7.STAT":u8)
    n648 = feedback #33(bool[] [FALSE, FALSE]) -> (w1245:bool[])
    n649 = Or(x=w1239, y=w1245) -> (x .or. y?=w1232:bool[])
    n650 = Index Array(array=w1232, index=w1229) -> (element=w1233:bool)
    n651 = case shown="真" w1233 {
      selector: w1233 -> [w1520 _]
      tunnel: [w1520 w1522] -> w1231
      tunnel: w1228 -> [_ w1521]
      frame False {
      }
      frame True {
        n652 = xnode ("FIFO Write")("元素"=w1521, "超时"=0 ("Timeout")) -> ("超时？"=w1522:bool)  [unwired: 1 in, 1 out]
      }
    }
    n653 = Unbundle By Name(w1333) -> ("I2C.DATI"=→"I2C.B.DATI":u8, "I2C.STAT"=→"I2C.B.STAT":u8)
    n654 = Replace Array Subset(array=w1232, new element=w1231, index=w1229) -> (w1230:bool[])
    n655 = feedback-in #33(w1230) -> ()
    n656 = call "Join Bank DIO.vi"("IN 7:4"=w1273, "IN 3:2"=w1274, "IN 1:0"=w1275, "IN 9:8"=w1272, "IN 11:10"=w1271, "IN 13:12"=w1270, "IN 15:14"=w1269, "IN 17:16"=w1268, "IN 19:18"=w1267) -> ("OUT 19:0"=w1276:fxp<+,20,20>)  [unwired: 6 in]
    n657 = xnode "FPGA I/O Node"() -> ("错误输出"=w1224:errorcluster)  [unwired: 2 in, 2 out]
    n658 = call "DIO Read Bank.vi"("DI.DMA_ENA"="DI.B.DMA_ENA", "DI.DMA_CNTR"="DI.B.DMA_CNTR", "DATA IN"=w1276, "DMA FIFO IN"=refnum<k21> "DI.B.DMA" ("FIFO")) -> ("DI.DMA_IDL"=→"DI.B.DMA_IDL":bool, "DIO.A_0:15.IN"=→"DIO.B_19:0.IN":fxp<+,20,20>)  [unwired: 6 in]
    n659 = Unbundle By Name(w1224) -> ("status"=→"UART.B.STAT":bool)
  }
  n660 = xnode "VI-Defined FIFO Configuration"() -> ()  [unwired: 1 out]
  n661 = node-c288(w19) -> ()
  n662 = while {
    stop <- FALSE stop-if-true
    # "The property node would allow user to explicitly enable or disable UART, so the user would already know if it is in UART mode or DIO mode."
    # "Set UART Enable Property"
    n663 = xnode "FPGA I/O Property Node"("ConnectorA - Uart Enable"="UART.A.ENA", "ConnectorB - Uart Enable"="UART.B.ENA") -> ("Console Out Enable"=→"CONSOLE.ENA":bool)  [unwired: 1 in, 1 out]
  }
